vi "DIALOG_Class Selection.vi"(7 "Action":T3=enum."Class For Node", 8 "Error In":errorcluster, 9 "User VI Ref":refnum<vi>, 10 "Class Name In":string, 11 "Classes":T4(array[cluster])=[{"Class Info"={"Unique ID string"="1", "Parent ID string"="", "Class Name (unlocalized)"="Application", "Class Name (localized)"="Application"}, "Class Heirarchy"="Application", "Class Type"=enum."Base", "Indent"=0}, {"Class Info"={"Unique ID string"="98", "Parent ID string"="", "Class Name (unlocalized)"="CopyConflict", "Class Name (localized)"="CopyConflict"}, "Class Heirarchy"="CopyConflict", "Class Type"=enum."Private", "Indent"=0}, {"Class Info"={"Unique ID string"="99", "Parent ID string"="", "Class Name (unlocalized)"="CopyExpert", "Class Name (localized)"="CopyExpert"}, "Class Heirarchy"="CopyExpert", "Class Type"=enum."Private", "Indent"=0}, {"Class Info"={"Unique ID string"="97", "Parent ID string"="", "Class Name (unlocalized)"="CopyItem", "Class Name (localized)"="CopyItem"}, "Class Heirarchy"="CopyItem", "Class Type"=enum."Private", "Indent"=0}, {"Class Info"={"Unique ID string"="94", "Parent ID string"="", "Class Name (unlocalized)"="CopyOperation", "Class Name (localized)"="CopyOperation"}, "Class Heirarchy"="CopyOperation", "Class Type"=enum."Private", "Indent"=0}, {"Class Info"={"Unique ID string"="3", "Parent ID string"="", "Class Name (unlocalized)"="Generic", "Class Name (localized)"="Generic"}, "Class Heirarchy"="Generic", "Class Type"=enum."Base", "Indent"=0}, {"Class Info"={"Unique ID string"="131", "Parent ID string"="3", "Class Name (unlocalized)"="Bus", "Class Name (localized)"="Bus"}, "Class Heirarchy"="Generic.Bus", "Class Type"=enum."Base", "Indent"=1}, {"Class Info"={"Unique ID string"="56", "Parent ID string"="3", "Class Name (unlocalized)"="ConnectorPane", "Class Name (localized)"="ConnectorPane"}, "Class Heirarchy"="Generic.ConnectorPane", "Class Type"=enum."Scripting", "Indent"=1}, {"Class Info"={"Unique ID string"="38", "Parent ID string"="3", "Class Name (unlocalized)"="Cursor", "Class Name (localized)"="Cursor"}, "Class Heirarchy"="Generic.Cursor", "Class Type"=enum."Base", "Indent"=1}, {"Class Info"={"Unique ID string"="16479", "Parent ID string"="3", "Class Name (unlocalized)"="FlatSequenceFrame", "Class Name (localized)"="FlatSequenceFrame"}, "Class Heirarchy"="Generic.FlatSequenceFrame", "Class Type"=enum."Scripting", "Indent"=1}, {"Class Info"={"Unique ID string"="16494", "Parent ID string"="16479", "Class Name (unlocalized)"="TimeSequenceFrame", "Class Name (localized)"="TimeSequenceFrame"}, "Class Heirarchy"="Generic.FlatSequenceFrame.TimeSequenceFrame", "Class Type"=enum."Scripting", "Indent"=2}, {"Class Info"={"Unique ID string"="36", "Parent ID string"="3", "Class Name (unlocalized)"="GObject", "Class Name (localized)"="GObject"}, "Class Heirarchy"="Generic.GObject", "Class Type"=enum."Base", "Indent"=1}, {"Class Info"={"Unique ID string"="16503", "Parent ID string"="36", "Class Name (unlocalized)"="AbstractDiagram", "Class Name (localized)"="AbstractDiagram"}, "Class Heirarchy"="Generic.GObject.AbstractDiagram", "Class Type"=enum."Scripting", "Indent"=2}, {"Class Info"={"Unique ID string"="16384", "Parent ID string"="16503", "Class Name (unlocalized)"="Diagram", "Class Name (localized)"="Diagram"}, "Class Heirarchy"="Generic.GObject.AbstractDiagram.Diagram", "Class Type"=enum."Scripting", "Indent"=3}, {"Class Info"={"Unique ID string"="16473", "Parent ID string"="16384", "Class Name (unlocalized)"="CompanionDiagram", "Class Name (localized)"="CompanionDiagram"}, "Class Heirarchy"="Generic.GObject.AbstractDiagram.Diagram.CompanionDiagram", "Class Type"=enum."Scripting", "Indent"=4}, {"Class Info"={"Unique ID string"="16489", "Parent ID string"="16384", "Class Name (unlocalized)"="SDF Companion Diagram", "Class Name (localized)"="SDF Companion Diagram"}, "Class Heirarchy"="Generic.GObject.AbstractDiagram.Diagram.SDF Companion Diagram", "Class Type"=enum."Scripting", "Indent"=4}, {"Class Info"={"Unique ID string"="16488", "Parent ID string"="16384", "Class Name (unlocalized)"="SDFDiagram", "Class Name (localized)"="SDFDiagram"}, "Class Heirarchy"="Generic.GObject.AbstractDiagram.Diagram.SDFDiagram", "Class Type"=enum."Scripting", "Indent"=4}, {"Class Info"={"Unique ID string"="16511", "Parent ID string"="16384", "Class Name (unlocalized)"="ScDiagram", "Class Name (localized)"="ScDiagram"}, "Class Heirarchy"="Generic.GObject.AbstractDiagram.Diagram.ScDiagram", "Class Type"=enum."Scripting", "Indent"=4}, {"Class Info"={"Unique ID string"="16472", "Parent ID string"="16384", "Class Name (unlocalized)"="SimDiagram", "Class Name (localized)"="SimDiagram"}, "Class Heirarchy"="Generic.GObject.AbstractDiagram.Diagram.SimDiagram", "Class Type"=enum."Scripting", "Indent"=4}, {"Class Info"={"Unique ID string"="16423", "Parent ID string"="16384", "Class Name (unlocalized)"="TopLevelDiagram", "Class Name (localized)"="TopLevelDiagram"}, "Class Heirarchy"="Generic.GObject.AbstractDiagram.Diagram.TopLevelDiagram", "Class Type"=enum."Scripting", "Indent"=4}, {"Class Info"={"Unique ID string"="16502", "Parent ID string"="16503", "Class Name (unlocalized)"="MathDiagram", "Class Name (localized)"="MathDiagram"}, "Class Heirarchy"="Generic.GObject.AbstractDiagram.MathDiagram", "Class Type"=enum."Scripting", "Indent"=3}, {"Class Info"={"Unique ID string"="16386", "Parent ID string"="36", "Class Name (unlocalized)"="Constant", "Class Name (localized)"="Constant"}, "Class Heirarchy"="Generic.GObject.Constant", "Class Type"=enum."Scripting", "Indent"=2}, {"Class Info"={"Unique ID string"="16461", "Parent ID string"="16386", "Class Name (unlocalized)"="AbsTimeConstant", "Class Name (localized)"="AbsTimeConstant"}, "Class Heirarchy"="Generic.GObject.Constant.AbsTimeConstant", "Class Type"=enum."Scripting", "Indent"=3}, {"Class Info"={"Unique ID string"="16388", "Parent ID string"="16386", "Class Name (unlocalized)"="ArrayConstant", "Class Name (localized)"="ArrayConstant"}, "Class Heirarchy"="Generic.GObject.Constant.ArrayConstant", "Class Type"=enum."Scripting", "Indent"=3}, {"Class Info"={"Unique ID string"="16422", "Parent ID string"="16386", "Class Name (unlocalized)"="BooleanConstant", "Class Name (localized)"="BooleanConstant"}, "Class Heirarchy"="Generic.GObject.Constant.BooleanConstant", "Class Type"=enum."Scripting", "Indent"=3}, {"Class Info"={"Unique ID string"="16393", "Parent ID string"="16386", "Class Name (unlocalized)"="ClusterConstant", "Class Name (localized)"="ClusterConstant"}, "Class Heirarchy"="Generic.GObject.Constant.ClusterConstant", "Class Type"=enum."Scripting", "Indent"=3}, {"Class Info"={"Unique ID string"="16450", "Parent ID string"="16386", "Class Name (unlocalized)"="ColorBoxConstant", "Class Name (localized)"="ColorBoxConstant"}, "Class Heirarchy"="Generic.GObject.Constant.ColorBoxConstant", "Class Type"=enum."Scripting", "Indent"=3}, {"Class Info"={"Unique ID string"="16394", "Parent ID string"="16386", "Class Name (unlocalized)"="FixedConstant", "Class Name (localized)"="FixedConstant"}, "Class Heirarchy"="Generic.GObject.Constant.FixedConstant", "Class Type"=enum."Scripting", "Indent"=3}, {"Class Info"={"Unique ID string"="16445", "Parent ID string"="16386", "Class Name (unlocalized)"="IONameConstant", "Class Name (localized)"="IONameConstant"}, "Class Heirarchy"="Generic.GObject.Constant.IONameConstant", "Class Type"=enum."Scripting", "Indent"=3}, {"Class Info"={"Unique ID string"="16447", "Parent ID string"="16445", "Class Name (unlocalized)"="DAQChannelNameConstant", "Class Name (localized)"="DAQChannelNameConstant"}, "Class Heirarchy"="Generic.GObject.Constant.IONameConstant.DAQChannelNameConstant", "Class Type"=enum."Scripting", "Indent"=4}, {"Class Info"={"Unique ID string"="16457", "Parent ID string"="16445", "Class Name (unlocalized)"="DAQmxNameConstant", "Class Name (localized)"="DAQmxNameConstant"}, "Class Heirarchy"="Generic.GObject.Constant.IONameConstant.DAQmxNameConstant", "Class Type"=enum."Scripting", "Indent"=4}, {"Class Info"={"Unique ID string"="16446", "Parent ID string"="16445", "Class Name (unlocalized)"="DSCTagConstant", "Class Name (localized)"="DSCTagConstant"}, "Class Heirarchy"="Generic.GObject.Constant.IONameConstant.DSCTagConstant", "Class Type"=enum."Scripting", "Indent"=4}, {"Class Info"={"Unique ID string"="16470", "Parent ID string"="16445", "Class Name (unlocalized)"="GenClassTagFlatRefConstant", "Class Name (localized)"="GenClassTagFlatRefConstant"}, "Class Heirarchy"="Generic.GObject.Constant.IONameConstant.GenClassTagFlatRefConstant", "Class Type"=enum."Scripting", "Indent"=4}, {"Class Info"={"Unique ID string"="16460", "Parent ID string"="16445", "Class Name (unlocalized)"="GenClassTagRefConstant", "Class Name (localized)"="GenClassTagRefConstant"}, "Class Heirarchy"="Generic.GObject.Constant.IONameConstant.GenClassTagRefConstant", "Class Type"=enum."Scripting", "Indent"=4}, {"Class Info"={"Unique ID string"="16449", "Parent ID string"="16445", "Class Name (unlocalized)"="IVILogicalNameConstant", "Class Name (localized)"="IVILogicalNameConstant"}, "Class Heirarchy"="Generic.GObject.Constant.IONameConstant.IVILogicalNameConstant", "Class Type"=enum."Scripting", "Indent"=4}, {"Class Info"={"Unique ID string"="16448", "Parent ID string"="16445", "Class Name (unlocalized)"="VISAResourceNameConstant", "Class Name (localized)"="VISAResourceNameConstant"}, "Class Heirarchy"="Generic.GObject.Constant.IONameConstant.VISAResourceNameConstant", "Class Type"=enum."Scripting", "Indent"=4}, {"Class Info"={"Unique ID string"="16501", "Parent ID string"="16386", "Class Name (unlocalized)"="LabVIEWClassConstant", "Class Name (localized)"="LabVIEWClassConstant"}, "Class Heirarchy"="Generic.GObject.Constant.LabVIEWClassConstant", "Class Type"=enum."Scripting", "Indent"=3}, {"Class Info"={"Unique ID string"="16553", "Parent ID string"="16386", "Class Name (unlocalized)"="MapConstant", "Class Name (localized)"="MapConstant"}, "Class Heirarchy"="Generic.GObject.Constant.MapConstant", "Class Type"=enum."Scripting", "Indent"=3}, {"Class Info"={"Unique ID string"="16389", "Parent ID string"="16386", "Class Name (unlocalized)"="NumericConstant", "Class Name (localized)"="NumericConstant"}, "Class Heirarchy"="Generic.GObject.Constant.NumericConstant", "Class Type"=enum."Scripting", "Indent"=3}, {"Class Info"={"Unique ID string"="16390", "Parent ID string"="16389", "Class Name (unlocalized)"="DigitalNumericConstant", "Class Name (localized)"="DigitalNumericConstant"}, "Class Heirarchy"="Generic.GObject.Constant.NumericConstant.DigitalNumericConstant", "Class Type"=enum."Scripting", "Indent"=4}, {"Class Info"={"Unique ID string"="16391", "Parent ID string"="16389", "Class Name (unlocalized)"="NamedNumericConstant", "Class Name (localized)"="NamedNumericConstant"}, "Class Heirarchy"="Generic.GObject.Constant.NumericConstant.NamedNumericConstant", "Class Type"=enum."Scripting", "Indent"=4}, {"Class Info"={"Unique ID string"="16425", "Parent ID string"="16391", "Class Name (unlocalized)"="EnumConstant", "Class Name (localized)"="EnumConstant"}, "Class Heirarchy"="Generic.GObject.Constant.NumericConstant.NamedNumericConstant.EnumConstant", "Class Type"=enum."Scripting", "Indent"=5}, {"Class Info"={"Unique ID string"="16424", "Parent ID string"="16391", "Class Name (unlocalized)"="RingConstant", "Class Name (localized)"="RingConstant"}, "Class Heirarchy"="Generic.GObject.Constant.NumericConstant.NamedNumericConstant.RingConstant", "Class Type"=enum."Scripting", "Indent"=5}, {"Class Info"={"Unique ID string"="16387", "Parent ID string"="16386", "Class Name (unlocalized)"="PathConstant", "Class Name (localized)"="PathConstant"}, "Class Heirarchy"="Generic.GObject.Constant.PathConstant", "Class Type"=enum."Scripting", "Indent"=3}, {"Class Info"={"Unique ID string"="16482", "Parent ID string"="16386", "Class Name (unlocalized)"="RefNumConstant", "Class Name (localized)"="RefNumConstant"}, "Class Heirarchy"="Generic.GObject.Constant.RefNumConstant", "Class Type"=enum."Scripting", "Indent"=3}, {"Class Info"={"Unique ID string"="16452", "Parent ID string"="16482", "Class Name (unlocalized)"="ClassSpecifierConstant", "Class Name (localized)"="ClassSpecifierConstant"}, "Class Heirarchy"="Generic.GObject.Constant.RefNumConstant.ClassSpecifierConstant", "Class Type"=enum."Scripting", "Indent"=4}, {"Class Info"={"Unique ID string"="16529", "Parent ID string"="16482", "Class Name (unlocalized)"="GenClassRefConst", "Class Name (localized)"="GenClassRefConst"}, "Class Heirarchy"="Generic.GObject.Constant.RefNumConstant.GenClassRefConst", "Class Type"=enum."Scripting", "Indent"=4}, {"Class Info"={"Unique ID string"="16538", "Parent ID string"="16482", "Class Name (unlocalized)"="TypedRefNumConstant", "Class Name (localized)"="TypedRefNumConstant"}, "Class Heirarchy"="Generic.GObject.Constant.RefNumConstant.TypedRefNumConstant", "Class Type"=enum."Scripting", "Indent"=4}, {"Class Info"={"Unique ID string"="16539", "Parent ID string"="16538", "Class Name (unlocalized)"="DataValRefNumConstant", "Class Name (localized)"="DataValRefNumConstant"}, "Class Heirarchy"="Generic.GObject.Constant.RefNumConstant.TypedRefNumConstant.DataValRefNumConstant", "Class Type"=enum."Scripting", "Indent"=5}, {"Class Info"={"Unique ID string"="16552", "Parent ID string"="16386", "Class Name (unlocalized)"="SetConstant", "Class Name (localized)"="SetConstant"}, "Class Heirarchy"="Generic.GObject.Constant.SetConstant", "Class Type"=enum."Scripting", "Indent"=3}, {"Class Info"={"Unique ID string"="16392", "Parent ID string"="16386", "Class Name (unlocalized)"="StringConstant", "Class Name (localized)"="StringConstant"}, "Class Heirarchy"="Generic.GObject.Constant.StringConstant", "Class Type"=enum."Scripting", "Indent"=3}, {"Class Info"={"Unique ID string"="16466", "Parent ID string"="16392", "Class Name (unlocalized)"="ComboBoxConstant", "Class Name (localized)"="ComboBoxConstant"}, "Class Heirarchy"="Generic.GObject.Constant.StringConstant.ComboBoxConstant", "Class Type"=enum."Scripting", "Indent"=4}, {"Class Info"={"Unique ID string"="6", "Parent ID string"="36", "Class Name (unlocalized)"="Control", "Class Name (localized)"="Control"}, "Class Heirarchy"="Generic.GObject.Control", "Class Type"=enum."Base", "Indent"=2}, {"Class Info"={"Unique ID string"="60", "Parent ID string"="6", "Class Name (unlocalized)"="AbsTime", "Class Name (localized)"="AbsTime"}, "Class Heirarchy"="Generic.GObject.Control.AbsTime", "Class Type"=enum."Base", "Indent"=3}, {"Class Info"={"Unique ID string"="16", "Parent ID string"="6", "Class Name (unlocalized)"="ActiveXContainer", "Class Name (localized)"="ActiveXContainer"}, "Class Heirarchy"="Generic.GObject.Control.ActiveXContainer", "Class Type"=enum."Base", "Indent"=3}, {"Class Info"={"Unique ID string"="14", "Parent ID string"="6", "Class Name (unlocalized)"="Array", "Class Name (localized)"="Array"}, "Class Heirarchy"="Generic.GObject.Control.Array", "Class Type"=enum."Base", "Indent"=3}, {"Class Info"={"Unique ID string"="8", "Parent ID string"="6", "Class Name (unlocalized)"="Boolean", "Class Name (localized)"="Boolean"}, "Class Heirarchy"="Generic.GObject.Control.Boolean", "Class Type"=enum."Base", "Indent"=3}, {"Class Info"={"Unique ID string"="30", "Parent ID string"="6", "Class Name (unlocalized)"="Cluster", "Class Name (localized)"="Cluster"}, "Class Heirarchy"="Generic.GObject.Control.Cluster", "Class Type"=enum."Base", "Indent"=3}, {"Class Info"={"Unique ID string"="72", "Parent ID string"="30", "Class Name (unlocalized)"="RadioButtonsControl", "Class Name (localized)"="RadioButtonsControl"}, "Class Heirarchy"="Generic.GObject.Control.Cluster.RadioButtonsControl", "Class Type"=enum."Base", "Indent"=4}, {"Class Info"={"Unique ID string"="7", "Parent ID string"="6", "Class Name (unlocalized)"="ColorBox", "Class Name (localized)"="ColorBox"}, "Class Heirarchy"="Generic.GObject.Control.ColorBox", "Class Type"=enum."Base", "Indent"=3}, {"Class Info"={"Unique ID string"="61", "Parent ID string"="6", "Class Name (unlocalized)"="DigitalTable", "Class Name (localized)"="DigitalTable"}, "Class Heirarchy"="Generic.GObject.Control.DigitalTable", "Class Type"=enum."Base", "Indent"=3}, {"Class Info"={"Unique ID string"="22", "Parent ID string"="6", "Class Name (unlocalized)"="GraphChart", "Class Name (localized)"="GraphChart"}, "Class Heirarchy"="Generic.GObject.Control.GraphChart", "Class Type"=enum."Base", "Indent"=3}, {"Class Info"={"Unique ID string"="25", "Parent ID string"="22", "Class Name (unlocalized)"="IntensityChart", "Class Name (localized)"="IntensityChart"}, "Class Heirarchy"="Generic.GObject.Control.GraphChart.IntensityChart", "Class Type"=enum."Base", "Indent"=4}, {"Class Info"={"Unique ID string"="26", "Parent ID string"="22", "Class Name (unlocalized)"="IntensityGraph", "Class Name (localized)"="IntensityGraph"}, "Class Heirarchy"="Generic.GObject.Control.GraphChart.IntensityGraph", "Class Type"=enum."Base", "Indent"=4}, {"Class Info"={"Unique ID string"="92", "Parent ID string"="22", "Class Name (unlocalized)"="MixedSignalGraph", "Class Name (localized)"="MixedSignalGraph"}, "Class Heirarchy"="Generic.GObject.Control.GraphChart.MixedSignalGraph", "Class Type"=enum."Base", "Indent"=4}, {"Class Info"={"Unique ID string"="23", "Parent ID string"="22", "Class Name (unlocalized)"="WaveformChart", "Class Name (localized)"="WaveformChart"}, "Class Heirarchy"="Generic.GObject.Control.GraphChart.WaveformChart", "Class Type"=enum."Base", "Indent"=4}, {"Class Info"={"Unique ID string"="24", "Parent ID string"="22", "Class Name (unlocalized)"="WaveformGraph", "Class Name (localized)"="WaveformGraph"}, "Class Heirarchy"="Generic.GObject.Control.GraphChart.WaveformGraph", "Class Type"=enum."Base", "Indent"=4}, {"Class Info"={"Unique ID string"="121", "Parent ID string"="24", "Class Name (unlocalized)"="DigitalGraph", "Class Name (localized)"="DigitalGraph"}, "Class Heirarchy"="Generic.GObject.Control.GraphChart.WaveformGraph.DigitalGraph", "Class Type"=enum."Base", "Indent"=5}, {"Class Info"={"Unique ID string"="83", "Parent ID string"="24", "Class Name (unlocalized)"="XYGraph", "Class Name (localized)"="XYGraph"}, "Class Heirarchy"="Generic.GObject.Control.GraphChart.WaveformGraph.XYGraph", "Class Type"=enum."Base", "Indent"=5}, {"Class Info"={"Unique ID string"="28", "Parent ID string"="6", "Class Name (unlocalized)"="IOName", "Class Name (localized)"="IOName"}, "Class Heirarchy"="Generic.GObject.Control.IOName", "Class Type"=enum."Base", "Indent"=3}, {"Class Info"={"Unique ID string"="49", "Parent ID string"="28", "Class Name (unlocalized)"="DAQChannelName", "Class Name (localized)"="DAQChannelName"}, "Class Heirarchy"="Generic.GObject.Control.IOName.DAQChannelName", "Class Type"=enum."Base", "Indent"=4}, {"Class Info"={"Unique ID string"="57", "Parent ID string"="28", "Class Name (unlocalized)"="DAQmxName", "Class Name (localized)"="DAQmxName"}, "Class Heirarchy"="Generic.GObject.Control.IOName.DAQmxName", "Class Type"=enum."Base", "Indent"=4}, {"Class Info"={"Unique ID string"="48", "Parent ID string"="28", "Class Name (unlocalized)"="DSCTag", "Class Name (localized)"="DSCTag"}, "Class Heirarchy"="Generic.GObject.Control.IOName.DSCTag", "Class Type"=enum."Base", "Indent"=4}, {"Class Info"={"Unique ID string"="122", "Parent ID string"="28", "Class Name (unlocalized)"="GenClassTagFlatRef", "Class Name (localized)"="GenClassTagFlatRef"}, "Class Heirarchy"="Generic.GObject.Control.IOName.GenClassTagFlatRef", "Class Type"=enum."Base", "Indent"=4}, {"Class Info"={"Unique ID string"="67", "Parent ID string"="28", "Class Name (unlocalized)"="GenClassTagRef", "Class Name (localized)"="GenClassTagRef"}, "Class Heirarchy"="Generic.GObject.Control.IOName.GenClassTagRef", "Class Type"=enum."Base", "Indent"=4}, {"Class Info"={"Unique ID string"="51", "Parent ID string"="28", "Class Name (unlocalized)"="IVILogicalName", "Class Name (localized)"="IVILogicalName"}, "Class Heirarchy"="Generic.GObject.Control.IOName.IVILogicalName", "Class Type"=enum."Base", "Indent"=4}, {"Class Info"={"Unique ID string"="50", "Parent ID string"="28", "Class Name (unlocalized)"="VISAResourceName", "Class Name (localized)"="VISAResourceName"}, "Class Heirarchy"="Generic.GObject.Control.IOName.VISAResourceName", "Class Type"=enum."Base", "Indent"=4}, {"Class Info"={"Unique ID string"="10", "Parent ID string"="6", "Class Name (unlocalized)"="LVVariant", "Class Name (localized)"="LVVariant"}, "Class Heirarchy"="Generic.GObject.Control.LVVariant", "Class Type"=enum."Base", "Indent"=3}, {"Class Info"={"Unique ID string"="102", "Parent ID string"="6", "Class Name (unlocalized)"="LabVIEWClassControl", "Class Name (localized)"="LabVIEWClassControl"}, "Class Heirarchy"="Generic.GObject.Control.LabVIEWClassControl", "Class Type"=enum."Base", "Indent"=3}, {"Class Info"={"Unique ID string"="12", "Parent ID string"="6", "Class Name (unlocalized)"="ListBox", "Class Name (localized)"="ListBox"}, "Class Heirarchy"="Generic.GObject.Control.ListBox", "Class Type"=enum."Base", "Indent"=3}, {"Class Info"={"Unique ID string"="137", "Parent ID string"="6", "Class Name (unlocalized)"="Map", "Class Name (localized)"="Map"}, "Class Heirarchy"="Generic.GObject.Control.Map", "Class Type"=enum."Base", "Indent"=3}, {"Class Info"={"Unique ID string"="127", "Parent ID string"="6", "Class Name (unlocalized)"="MixedCheckbox", "Class Name (localized)"="MixedCheckbox"}, "Class Heirarchy"="Generic.GObject.Control.MixedCheckbox", "Class Type"=enum."Base", "Indent"=3}, {"Class Info"={"Unique ID string"="130", "Parent ID string"="6", "Class Name (unlocalized)"="MultiSegmentPipe", "Class Name (localized)"="MultiSegmentPipe"}, "Class Heirarchy"="Generic.GObject.Control.MultiSegmentPipe", "Class Type"=enum."Base", "Indent"=3}, {"Class Info"={"Unique ID string"="46", "Parent ID string"="6", "Class Name (unlocalized)"="MulticolumnListbox", "Class Name (localized)"="MulticolumnListbox"}, "Class Heirarchy"="Generic.GObject.Control.MulticolumnListbox", "Class Type"=enum."Base", "Indent"=3}, {"Class Info"={"Unique ID string"="17", "Parent ID string"="6", "Class Name (unlocalized)"="Numeric", "Class Name (localized)"="Numeric"}, "Class Heirarchy"="Generic.GObject.Control.Numeric", "Class Type"=enum."Base", "Indent"=3}, {"Class Info"={"Unique ID string"="20", "Parent ID string"="17", "Class Name (unlocalized)"="ColorRamp", "Class Name (localized)"="ColorRamp"}, "Class Heirarchy"="Generic.GObject.Control.Numeric.ColorRamp", "Class Type"=enum."Base", "Indent"=4}, {"Class Info"={"Unique ID string"="18", "Parent ID string"="17", "Class Name (unlocalized)"="Digital", "Class Name (localized)"="Digital"}, "Class Heirarchy"="Generic.GObject.Control.Numeric.Digital", "Class Type"=enum."Base", "Indent"=4}, {"Class Info"={"Unique ID string"="19", "Parent ID string"="17", "Class Name (unlocalized)"="NamedNumeric", "Class Name (localized)"="NamedNumeric"}, "Class Heirarchy"="Generic.GObject.Control.Numeric.NamedNumeric", "Class Type"=enum."Base", "Indent"=4}, {"Class Info"={"Unique ID string"="35", "Parent ID string"="19", "Class Name (unlocalized)"="Enum", "Class Name (localized)"="Enum"}, "Class Heirarchy"="Generic.GObject.Control.Numeric.NamedNumeric.Enum", "Class Type"=enum."Base", "Indent"=5}, {"Class Info"={"Unique ID string"="34", "Parent ID string"="19", "Class Name (unlocalized)"="Ring", "Class Name (localized)"="Ring"}, "Class Heirarchy"="Generic.GObject.Control.Numeric.NamedNumeric.Ring", "Class Type"=enum."Base", "Indent"=5}, {"Class Info"={"Unique ID string"="33", "Parent ID string"="17", "Class Name (unlocalized)"="NumericWithScale", "Class Name (localized)"="NumericWithScale"}, "Class Heirarchy"="Generic.GObject.Control.Numeric.NumericWithScale", "Class Type"=enum."Base", "Indent"=4}, {"Class Info"={"Unique ID string"="32", "Parent ID string"="33", "Class Name (unlocalized)"="Knob", "Class Name (localized)"="Knob"}, "Class Heirarchy"="Generic.GObject.Control.Numeric.NumericWithScale.Knob", "Class Type"=enum."Base", "Indent"=5}, {"Class Info"={"Unique ID string"="21", "Parent ID string"="33", "Class Name (unlocalized)"="Slide", "Class Name (localized)"="Slide"}, "Class Heirarchy"="Generic.GObject.Control.Numeric.NumericWithScale.Slide", "Class Type"=enum."Base", "Indent"=5}, {"Class Info"={"Unique ID string"="53", "Parent ID string"="6", "Class Name (unlocalized)"="PageSelector", "Class Name (localized)"="PageSelector"}, "Class Heirarchy"="Generic.GObject.Control.PageSelector", "Class Type"=enum."Base", "Indent"=3}, {"Class Info"={"Unique ID string"="55", "Parent ID string"="53", "Class Name (unlocalized)"="TabControl", "Class Name (localized)"="TabControl"}, "Class Heirarchy"="Generic.GObject.Control.PageSelector.TabControl", "Class Type"=enum."Base", "Indent"=4}, {"Class Info"={"Unique ID string"="11", "Parent ID string"="6", "Class Name (unlocalized)"="Path", "Class Name (localized)"="Path"}, "Class Heirarchy"="Generic.GObject.Control.Path", "Class Type"=enum."Base", "Indent"=3}, {"Class Info"={"Unique ID string"="15", "Parent ID string"="6", "Class Name (unlocalized)"="Picture", "Class Name (localized)"="Picture"}, "Class Heirarchy"="Generic.GObject.Control.Picture", "Class Type"=enum."Base", "Indent"=3}, {"Class Info"={"Unique ID string"="78", "Parent ID string"="6", "Class Name (unlocalized)"="Pixmap", "Class Name (localized)"="Pixmap"}, "Class Heirarchy"="Generic.GObject.Control.Pixmap", "Class Type"=enum."Base", "Indent"=3}, {"Class Info"={"Unique ID string"="70", "Parent ID string"="6", "Class Name (unlocalized)"="PlugInControl", "Class Name (localized)"="PlugInControl"}, "Class Heirarchy"="Generic.GObject.Control.PlugInControl", "Class Type"=enum."Base", "Indent"=3}, {"Class Info"={"Unique ID string"="71", "Parent ID string"="6", "Class Name (unlocalized)"="PlugInDDODummyContainer", "Class Name (localized)"="PlugInDDODummyContainer"}, "Class Heirarchy"="Generic.GObject.Control.PlugInDDODummyContainer", "Class Type"=enum."Base", "Indent"=3}, {"Class Info"={"Unique ID string"="9", "Parent ID string"="6", "Class Name (unlocalized)"="RefNum", "Class Name (localized)"="RefNum"}, "Class Heirarchy"="Generic.GObject.Control.RefNum", "Class Type"=enum."Base", "Indent"=3}, {"Class Info"={"Unique ID string"="68", "Parent ID string"="9", "Class Name (unlocalized)"="GenClassRef", "Class Name (localized)"="GenClassRef"}, "Class Heirarchy"="Generic.GObject.Control.RefNum.GenClassRef", "Class Type"=enum."Base", "Indent"=4}, {"Class Info"={"Unique ID string"="59", "Parent ID string"="9", "Class Name (unlocalized)"="LVObjectRefNum", "Class Name (localized)"="LVObjectRefNum"}, "Class Heirarchy"="Generic.GObject.Control.RefNum.LVObjectRefNum", "Class Type"=enum."Base", "Indent"=4}, {"Class Info"={"Unique ID string"="58", "Parent ID string"="59", "Class Name (unlocalized)"="VIRefNum", "Class Name (localized)"="VIRefNum"}, "Class Heirarchy"="Generic.GObject.Control.RefNum.LVObjectRefNum.VIRefNum", "Class Type"=enum."Base", "Indent"=5}, {"Class Info"={"Unique ID string"="44", "Parent ID string"="9", "Class Name (unlocalized)"="TypedRefNum", "Class Name (localized)"="TypedRefNum"}, "Class Heirarchy"="Generic.GObject.Control.RefNum.TypedRefNum", "Class Type"=enum."Base", "Indent"=4}, {"Class Info"={"Unique ID string"="135", "Parent ID string"="44", "Class Name (unlocalized)"="DataValRefNum", "Class Name (localized)"="DataValRefNum"}, "Class Heirarchy"="Generic.GObject.Control.RefNum.TypedRefNum.DataValRefNum", "Class Type"=enum."Base", "Indent"=5}, {"Class Info"={"Unique ID string"="100", "Parent ID string"="6", "Class Name (unlocalized)"="SceneGraphDisplay", "Class Name (localized)"="SceneGraphDisplay"}, "Class Heirarchy"="Generic.GObject.Control.SceneGraphDisplay", "Class Type"=enum."Base", "Indent"=3}, {"Class Info"={"Unique ID string"="90", "Parent ID string"="6", "Class Name (unlocalized)"="Scrollbar", "Class Name (localized)"="Scrollbar"}, "Class Heirarchy"="Generic.GObject.Control.Scrollbar", "Class Type"=enum."Base", "Indent"=3}, {"Class Info"={"Unique ID string"="136", "Parent ID string"="6", "Class Name (unlocalized)"="Set", "Class Name (localized)"="Set"}, "Class Heirarchy"="Generic.GObject.Control.Set", "Class Type"=enum."Base", "Indent"=3}, {"Class Info"={"Unique ID string"="27", "Parent ID string"="6", "Class Name (unlocalized)"="String", "Class Name (localized)"="String"}, "Class Heirarchy"="Generic.GObject.Control.String", "Class Type"=enum."Base", "Indent"=3}, {"Class Info"={"Unique ID string"="29", "Parent ID string"="27", "Class Name (unlocalized)"="ComboBox", "Class Name (localized)"="ComboBox"}, "Class Heirarchy"="Generic.GObject.Control.String.ComboBox", "Class Type"=enum."Base", "Indent"=4}, {"Class Info"={"Unique ID string"="132", "Parent ID string"="6", "Class Name (unlocalized)"="StubDDO", "Class Name (localized)"="StubDDO"}, "Class Heirarchy"="Generic.GObject.Control.StubDDO", "Class Type"=enum."Base", "Indent"=3}, {"Class Info"={"Unique ID string"="65", "Parent ID string"="6", "Class Name (unlocalized)"="SubPanel", "Class Name (localized)"="SubPanel"}, "Class Heirarchy"="Generic.GObject.Control.SubPanel", "Class Type"=enum."Base", "Indent"=3}, {"Class Info"={"Unique ID string"="13", "Parent ID string"="6", "Class Name (unlocalized)"="Table", "Class Name (localized)"="Table"}, "Class Heirarchy"="Generic.GObject.Control.Table", "Class Type"=enum."Base", "Indent"=3}, {"Class Info"={"Unique ID string"="66", "Parent ID string"="6", "Class Name (unlocalized)"="TreeControl", "Class Name (localized)"="TreeControl"}, "Class Heirarchy"="Generic.GObject.Control.TreeControl", "Class Type"=enum."Base", "Indent"=3}, {"Class Info"={"Unique ID string"="47", "Parent ID string"="6", "Class Name (unlocalized)"="WaveformData", "Class Name (localized)"="WaveformData"}, "Class Heirarchy"="Generic.GObject.Control.WaveformData", "Class Type"=enum."Base", "Indent"=3}, {"Class Info"={"Unique ID string"="4", "Parent ID string"="36", "Class Name (unlocalized)"="Decoration", "Class Name (localized)"="Decoration"}, "Class Heirarchy"="Generic.GObject.Decoration", "Class Type"=enum."Base", "Indent"=2}, {"Class Info"={"Unique ID string"="5", "Parent ID string"="4", "Class Name (unlocalized)"="Text", "Class Name (localized)"="Text"}, "Class Heirarchy"="Generic.GObject.Decoration.Text", "Class Type"=enum."Base", "Indent"=3}, {"Class Info"={"Unique ID string"="39", "Parent ID string"="5", "Class Name (unlocalized)"="NumericText", "Class Name (localized)"="NumericText"}, "Class Heirarchy"="Generic.GObject.Decoration.Text.NumericText", "Class Type"=enum."Base", "Indent"=4}, {"Class Info"={"Unique ID string"="16459", "Parent ID string"="36", "Class Name (unlocalized)"="FlatSequence", "Class Name (localized)"="FlatSequence"}, "Class Heirarchy"="Generic.GObject.FlatSequence", "Class Type"=enum."Scripting", "Indent"=2}, {"Class Info"={"Unique ID string"="16495", "Parent ID string"="16459", "Class Name (unlocalized)"="TimeFlatSequence", "Class Name (localized)"="TimeFlatSequence"}, "Class Heirarchy"="Generic.GObject.FlatSequence.TimeFlatSequence", "Class Type"=enum."Scripting", "Indent"=3}, {"Class Info"={"Unique ID string"="16480", "Parent ID string"="36", "Class Name (unlocalized)"="FlatSequenceInnerTunnel", "Class Name (localized)"="FlatSequenceInnerTunnel"}, "Class Heirarchy"="Generic.GObject.FlatSequenceInnerTunnel", "Class Type"=enum."Scripting", "Indent"=2}, {"Class Info"={"Unique ID string"="16481", "Parent ID string"="36", "Class Name (unlocalized)"="FlatSequenceOuterTunnel", "Class Name (localized)"="FlatSequenceOuterTunnel"}, "Class Heirarchy"="Generic.GObject.FlatSequenceOuterTunnel", "Class Type"=enum."Scripting", "Indent"=2}, {"Class Info"={"Unique ID string"="16396", "Parent ID string"="36", "Class Name (unlocalized)"="FormulaParameter", "Class Name (localized)"="FormulaParameter"}, "Class Heirarchy"="Generic.GObject.FormulaParameter", "Class Type"=enum."Scripting", "Indent"=2}, {"Class Info"={"Unique ID string"="16500", "Parent ID string"="16396", "Class Name (unlocalized)"="MathScriptNodeParameter", "Class Name (localized)"="MathScriptNodeParameter"}, "Class Heirarchy"="Generic.GObject.FormulaParameter.MathScriptNodeParameter", "Class Type"=enum."Scripting", "Indent"=3}, {"Class Info"={"Unique ID string"="16464", "Parent ID string"="16396", "Class Name (unlocalized)"="ScriptNodeParameter", "Class Name (localized)"="ScriptNodeParameter"}, "Class Heirarchy"="Generic.GObject.FormulaParameter.ScriptNodeParameter", "Class Type"=enum."Scripting", "Indent"=3}, {"Class Info"={"Unique ID string"="16421", "Parent ID string"="36", "Class Name (unlocalized)"="Node", "Class Name (localized)"="Node"}, "Class Heirarchy"="Generic.GObject.Node", "Class Type"=enum."Scripting", "Indent"=2}, {"Class Info"={"Unique ID string"="16402", "Parent ID string"="16421", "Class Name (unlocalized)"="CallByRef", "Class Name (localized)"="CallByRef"}, "Class Heirarchy"="Generic.GObject.Node.CallByRef", "Class Type"=enum."Scripting", "Indent"=3}, {"Class Info"={"Unique ID string"="16451", "Parent ID string"="16421", "Class Name (unlocalized)"="ControlReferenceConstant", "Class Name (localized)"="ControlReferenceConstant"}, "Class Heirarchy"="Generic.GObject.Node.ControlReferenceConstant", "Class Type"=enum."Scripting", "Indent"=3}, {"Class Info"={"Unique ID string"="16522", "Parent ID string"="16421", "Class Name (unlocalized)"="FeedbackNode", "Class Name (localized)"="FeedbackNode"}, "Class Heirarchy"="Generic.GObject.Node.FeedbackNode", "Class Type"=enum."Scripting", "Indent"=3}, {"Class Info"={"Unique ID string"="16409", "Parent ID string"="16421", "Class Name (unlocalized)"="Formula", "Class Name (localized)"="Formula"}, "Class Heirarchy"="Generic.GObject.Node.Formula", "Class Type"=enum."Scripting", "Indent"=3}, {"Class Info"={"Unique ID string"="16504", "Parent ID string"="16409", "Class Name (unlocalized)"="InlineCNode", "Class Name (localized)"="InlineCNode"}, "Class Heirarchy"="Generic.GObject.Node.Formula.InlineCNode", "Class Type"=enum."Scripting", "Indent"=4}, {"Class Info"={"Unique ID string"="16499", "Parent ID string"="16409", "Class Name (unlocalized)"="MathScriptNode", "Class Name (localized)"="MathScriptNode"}, "Class Heirarchy"="Generic.GObject.Node.Formula.MathScriptNode", "Class Type"=enum."Scripting", "Indent"=4}, {"Class Info"={"Unique ID string"="16436", "Parent ID string"="16409", "Class Name (unlocalized)"="ScriptNode", "Class Name (localized)"="ScriptNode"}, "Class Heirarchy"="Generic.GObject.Node.Formula.ScriptNode", "Class Type"=enum."Scripting", "Indent"=4}, {"Class Info"={"Unique ID string"="16400", "Parent ID string"="16421", "Class Name (unlocalized)"="Function", "Class Name (localized)"="Function"}, "Class Heirarchy"="Generic.GObject.Node.Function", "Class Type"=enum."Scripting", "Indent"=3}, {"Class Info"={"Unique ID string"="16437", "Parent ID string"="16400", "Class Name (unlocalized)"="ArrayToCluster", "Class Name (localized)"="ArrayToCluster"}, "Class Heirarchy"="Generic.GObject.Node.Function.ArrayToCluster", "Class Type"=enum."Scripting", "Indent"=4}, {"Class Info"={"Unique ID string"="16429", "Parent ID string"="16400", "Class Name (unlocalized)"="Comparison", "Class Name (localized)"="Comparison"}, "Class Heirarchy"="Generic.GObject.Node.Function.Comparison", "Class Type"=enum."Scripting", "Indent"=4}, {"Class Info"={"Unique ID string"="16535", "Parent ID string"="16429", "Class Name (unlocalized)"="InRangeAndCoerce", "Class Name (localized)"="InRangeAndCoerce"}, "Class Heirarchy"="Generic.GObject.Node.Function.Comparison.InRangeAndCoerce", "Class Type"=enum."Scripting", "Indent"=5}, {"Class Info"={"Unique ID string"="16492", "Parent ID string"="16400", "Class Name (unlocalized)"="FileDialog", "Class Name (localized)"="FileDialog"}, "Class Heirarchy"="Generic.GObject.Node.Function.FileDialog", "Class Type"=enum."Scripting", "Indent"=4}, {"Class Info"={"Unique ID string"="16432", "Parent ID string"="16400", "Class Name (unlocalized)"="FlattenUnflattenString", "Class Name (localized)"="FlattenUnflattenString"}, "Class Heirarchy"="Generic.GObject.Node.Function.FlattenUnflattenString", "Class Type"=enum."Scripting", "Indent"=4}, {"Class Info"={"Unique ID string"="16483", "Parent ID string"="16432", "Class Name (unlocalized)"="FlattenString", "Class Name (localized)"="FlattenString"}, "Class Heirarchy"="Generic.GObject.Node.Function.FlattenUnflattenString.FlattenString", "Class Type"=enum."Scripting", "Indent"=5}, {"Class Info"={"Unique ID string"="16433", "Parent ID string"="16400", "Class Name (unlocalized)"="GPIBReadWrite", "Class Name (localized)"="GPIBReadWrite"}, "Class Heirarchy"="Generic.GObject.Node.Function.GPIBReadWrite", "Class Type"=enum."Scripting", "Indent"=4}, {"Class Info"={"Unique ID string"="16430", "Parent ID string"="16400", "Class Name (unlocalized)"="ReadWriteFile", "Class Name (localized)"="ReadWriteFile"}, "Class Heirarchy"="Generic.GObject.Node.Function.ReadWriteFile", "Class Type"=enum."Scripting", "Indent"=4}, {"Class Info"={"Unique ID string"="16431", "Parent ID string"="16400", "Class Name (unlocalized)"="TypeCast", "Class Name (localized)"="TypeCast"}, "Class Heirarchy"="Generic.GObject.Node.Function.TypeCast", "Class Type"=enum."Scripting", "Indent"=4}, {"Class Info"={"Unique ID string"="16397", "Parent ID string"="16421", "Class Name (unlocalized)"="Global", "Class Name (localized)"="Global"}, "Class Heirarchy"="Generic.GObject.Node.Global", "Class Type"=enum."Scripting", "Indent"=3}, {"Class Info"={"Unique ID string"="16410", "Parent ID string"="16421", "Class Name (unlocalized)"="GrowableFunction", "Class Name (localized)"="GrowableFunction"}, "Class Heirarchy"="Generic.GObject.Node.GrowableFunction", "Class Type"=enum."Scripting", "Indent"=3}, {"Class Info"={"Unique ID string"="16551", "Parent ID string"="16410", "Class Name (unlocalized)"="AssertStructuralTypeMismatchNode", "Class Name (localized)"="AssertStructuralTypeMismatchNode"}, "Class Heirarchy"="Generic.GObject.Node.GrowableFunction.AssertStructuralTypeMismatchNode", "Class Type"=enum."Scripting", "Indent"=4}, {"Class Info"={"Unique ID string"="16411", "Parent ID string"="16410", "Class Name (unlocalized)"="BuildClusterArray", "Class Name (localized)"="BuildClusterArray"}, "Class Heirarchy"="Generic.GObject.Node.GrowableFunction.BuildClusterArray", "Class Type"=enum."Scripting", "Indent"=4}, {"Class Info"={"Unique ID string"="16550", "Parent ID string"="16410", "Class Name (unlocalized)"="BuildMapNode", "Class Name (localized)"="BuildMapNode"}, "Class Heirarchy"="Generic.GObject.Node.GrowableFunction.BuildMapNode", "Class Type"=enum."Scripting", "Indent"=4}, {"Class Info"={"Unique ID string"="16549", "Parent ID string"="16410", "Class Name (unlocalized)"="BuildSetNode", "Class Name (localized)"="BuildSetNode"}, "Class Heirarchy"="Generic.GObject.Node.GrowableFunction.BuildSetNode", "Class Type"=enum."Scripting", "Indent"=4}, {"Class Info"={"Unique ID string"="16476", "Parent ID string"="16410", "Class Name (unlocalized)"="Bundler", "Class Name (localized)"="Bundler"}, "Class Heirarchy"="Generic.GObject.Node.GrowableFunction.Bundler", "Class Type"=enum."Scripting", "Indent"=4}, {"Class Info"={"Unique ID string"="16414", "Parent ID string"="16476", "Class Name (unlocalized)"="BuildArray", "Class Name (localized)"="BuildArray"}, "Class Heirarchy"="Generic.GObject.Node.GrowableFunction.Bundler.BuildArray", "Class Type"=enum."Scripting", "Indent"=5}, {"Class Info"={"Unique ID string"="16415", "Parent ID string"="16476", "Class Name (unlocalized)"="NamedBundler", "Class Name (localized)"="NamedBundler"}, "Class Heirarchy"="Generic.GObject.Node.GrowableFunction.Bundler.NamedBundler", "Class Type"=enum."Scripting", "Indent"=5}, {"Class Info"={"Unique ID string"="16416", "Parent ID string"="16410", "Class Name (unlocalized)"="CIN", "Class Name (localized)"="CIN"}, "Class Heirarchy"="Generic.GObject.Node.GrowableFunction.CIN", "Class Type"=enum."Scripting", "Indent"=4}, {"Class Info"={"Unique ID string"="16417", "Parent ID string"="16410", "Class Name (unlocalized)"="CallLibrary", "Class Name (localized)"="CallLibrary"}, "Class Heirarchy"="Generic.GObject.Node.GrowableFunction.CallLibrary", "Class Type"=enum."Scripting", "Indent"=4}, {"Class Info"={"Unique ID string"="16412", "Parent ID string"="16410", "Class Name (unlocalized)"="CompoundArithmetic", "Class Name (localized)"="CompoundArithmetic"}, "Class Heirarchy"="Generic.GObject.Node.GrowableFunction.CompoundArithmetic", "Class Type"=enum."Scripting", "Indent"=4}, {"Class Info"={"Unique ID string"="16438", "Parent ID string"="16410", "Class Name (unlocalized)"="FormatScanString", "Class Name (localized)"="FormatScanString"}, "Class Heirarchy"="Generic.GObject.Node.GrowableFunction.FormatScanString", "Class Type"=enum."Scripting", "Indent"=4}, {"Class Info"={"Unique ID string"="16413", "Parent ID string"="16410", "Class Name (unlocalized)"="IndexArray", "Class Name (localized)"="IndexArray"}, "Class Heirarchy"="Generic.GObject.Node.GrowableFunction.IndexArray", "Class Type"=enum."Scripting", "Indent"=4}, {"Class Info"={"Unique ID string"="16418", "Parent ID string"="16410", "Class Name (unlocalized)"="ObjectFunction", "Class Name (localized)"="ObjectFunction"}, "Class Heirarchy"="Generic.GObject.Node.GrowableFunction.ObjectFunction", "Class Type"=enum."Scripting", "Indent"=4}, {"Class Info"={"Unique ID string"="16505", "Parent ID string"="16418", "Class Name (unlocalized)"="Constructor", "Class Name (localized)"="Constructor"}, "Class Heirarchy"="Generic.GObject.Node.GrowableFunction.ObjectFunction.Constructor", "Class Type"=enum."Scripting", "Indent"=5}, {"Class Info"={"Unique ID string"="16420", "Parent ID string"="16418", "Class Name (unlocalized)"="Invoke", "Class Name (localized)"="Invoke"}, "Class Heirarchy"="Generic.GObject.Node.GrowableFunction.ObjectFunction.Invoke", "Class Type"=enum."Scripting", "Indent"=5}, {"Class Info"={"Unique ID string"="16419", "Parent ID string"="16418", "Class Name (unlocalized)"="Property", "Class Name (localized)"="Property"}, "Class Heirarchy"="Generic.GObject.Node.GrowableFunction.ObjectFunction.Property", "Class Type"=enum."Scripting", "Indent"=5}, {"Class Info"={"Unique ID string"="16542", "Parent ID string"="16410", "Class Name (unlocalized)"="RegisterForEvents", "Class Name (localized)"="RegisterForEvents"}, "Class Heirarchy"="Generic.GObject.Node.GrowableFunction.RegisterForEvents", "Class Type"=enum."Scripting", "Indent"=4}, {"Class Info"={"Unique ID string"="16477", "Parent ID string"="16410", "Class Name (unlocalized)"="Unbundler", "Class Name (localized)"="Unbundler"}, "Class Heirarchy"="Generic.GObject.Node.GrowableFunction.Unbundler", "Class Type"=enum."Scripting", "Indent"=4}, {"Class Info"={"Unique ID string"="16478", "Parent ID string"="16477", "Class Name (unlocalized)"="NamedUnbundler", "Class Name (localized)"="NamedUnbundler"}, "Class Heirarchy"="Generic.GObject.Node.GrowableFunction.Unbundler.NamedUnbundler", "Class Type"=enum."Scripting", "Indent"=5}, {"Class Info"={"Unique ID string"="16517", "Parent ID string"="16421", "Class Name (unlocalized)"="InPlaceBorderNode", "Class Name (localized)"="InPlaceBorderNode"}, "Class Heirarchy"="Generic.GObject.Node.InPlaceBorderNode", "Class Type"=enum."Scripting", "Indent"=3}, {"Class Info"={"Unique ID string"="16518", "Parent ID string"="16517", "Class Name (unlocalized)"="InPlaceArrayNode", "Class Name (localized)"="InPlaceArrayNode"}, "Class Heirarchy"="Generic.GObject.Node.InPlaceBorderNode.InPlaceArrayNode", "Class Type"=enum."Scripting", "Indent"=4}, {"Class Info"={"Unique ID string"="16530", "Parent ID string"="16517", "Class Name (unlocalized)"="InPlaceArraySplitNode", "Class Name (localized)"="InPlaceArraySplitNode"}, "Class Heirarchy"="Generic.GObject.Node.InPlaceBorderNode.InPlaceArraySplitNode", "Class Type"=enum."Scripting", "Indent"=4}, {"Class Info"={"Unique ID string"="16519", "Parent ID string"="16517", "Class Name (unlocalized)"="InPlaceClusterNode", "Class Name (localized)"="InPlaceClusterNode"}, "Class Heirarchy"="Generic.GObject.Node.InPlaceBorderNode.InPlaceClusterNode", "Class Type"=enum."Scripting", "Indent"=4}, {"Class Info"={"Unique ID string"="16524", "Parent ID string"="16517", "Class Name (unlocalized)"="InPlaceDataValRefNode", "Class Name (localized)"="InPlaceDataValRefNode"}, "Class Heirarchy"="Generic.GObject.Node.InPlaceBorderNode.InPlaceDataValRefNode", "Class Type"=enum."Scripting", "Indent"=4}, {"Class Info"={"Unique ID string"="16521", "Parent ID string"="16517", "Class Name (unlocalized)"="InPlaceElementNode", "Class Name (localized)"="InPlaceElementNode"}, "Class Heirarchy"="Generic.GObject.Node.InPlaceBorderNode.InPlaceElementNode", "Class Type"=enum."Scripting", "Indent"=4}, {"Class Info"={"Unique ID string"="16548", "Parent ID string"="16517", "Class Name (unlocalized)"="InPlaceMapNode", "Class Name (localized)"="InPlaceMapNode"}, "Class Heirarchy"="Generic.GObject.Node.InPlaceBorderNode.InPlaceMapNode", "Class Type"=enum."Scripting", "Indent"=4}, {"Class Info"={"Unique ID string"="16544", "Parent ID string"="16517", "Class Name (unlocalized)"="InPlaceVariantAttributeNode", "Class Name (localized)"="InPlaceVariantAttributeNode"}, "Class Heirarchy"="Generic.GObject.Node.InPlaceBorderNode.InPlaceVariantAttributeNode", "Class Type"=enum."Scripting", "Indent"=4}, {"Class Info"={"Unique ID string"="16520", "Parent ID string"="16517", "Class Name (unlocalized)"="InPlaceVariantNode", "Class Name (localized)"="InPlaceVariantNode"}, "Class Heirarchy"="Generic.GObject.Node.InPlaceBorderNode.InPlaceVariantNode", "Class Type"=enum."Scripting", "Indent"=4}, {"Class Info"={"Unique ID string"="16398", "Parent ID string"="16421", "Class Name (unlocalized)"="Local", "Class Name (localized)"="Local"}, "Class Heirarchy"="Generic.GObject.Node.Local", "Class Type"=enum."Scripting", "Indent"=3}, {"Class Info"={"Unique ID string"="16523", "Parent ID string"="16421", "Class Name (unlocalized)"="MathScriptCallByRef", "Class Name (localized)"="MathScriptCallByRef"}, "Class Heirarchy"="Generic.GObject.Node.MathScriptCallByRef", "Class Type"=enum."Scripting", "Indent"=3}, {"Class Info"={"Unique ID string"="16531", "Parent ID string"="16421", "Class Name (unlocalized)"="SharedVariableDynamicOpen", "Class Name (localized)"="SharedVariableDynamicOpen"}, "Class Heirarchy"="Generic.GObject.Node.SharedVariableDynamicOpen", "Class Type"=enum."Scripting", "Indent"=3}, {"Class Info"={"Unique ID string"="16532", "Parent ID string"="16421", "Class Name (unlocalized)"="SharedVariableDynamicRead", "Class Name (localized)"="SharedVariableDynamicRead"}, "Class Heirarchy"="Generic.GObject.Node.SharedVariableDynamicRead", "Class Type"=enum."Scripting", "Indent"=3}, {"Class Info"={"Unique ID string"="16533", "Parent ID string"="16421", "Class Name (unlocalized)"="SharedVariableDynamicWrite", "Class Name (localized)"="SharedVariableDynamicWrite"}, "Class Heirarchy"="Generic.GObject.Node.SharedVariableDynamicWrite", "Class Type"=enum."Scripting", "Indent"=3}, {"Class Info"={"Unique ID string"="16512", "Parent ID string"="16421", "Class Name (unlocalized)"="SharedVariableNode", "Class Name (localized)"="SharedVariableNode"}, "Class Heirarchy"="Generic.GObject.Node.SharedVariableNode", "Class Type"=enum."Scripting", "Indent"=3}, {"Class Info"={"Unique ID string"="16465", "Parent ID string"="16421", "Class Name (unlocalized)"="StaticVIReference", "Class Name (localized)"="StaticVIReference"}, "Class Heirarchy"="Generic.GObject.Node.StaticVIReference", "Class Type"=enum."Scripting", "Indent"=3}, {"Class Info"={"Unique ID string"="16404", "Parent ID string"="16421", "Class Name (unlocalized)"="Structure", "Class Name (localized)"="Structure"}, "Class Heirarchy"="Generic.GObject.Node.Structure", "Class Type"=enum."Scripting", "Indent"=3}, {"Class Info"={"Unique ID string"="16545", "Parent ID string"="16404", "Class Name (unlocalized)"="ClosureStructureNode", "Class Name (localized)"="ClosureStructureNode"}, "Class Heirarchy"="Generic.GObject.Node.Structure.ClosureStructureNode", "Class Type"=enum."Scripting", "Indent"=4}, {"Class Info"={"Unique ID string"="16516", "Parent ID string"="16404", "Class Name (unlocalized)"="InPlaceElementStructure", "Class Name (localized)"="InPlaceElementStructure"}, "Class Heirarchy"="Generic.GObject.Node.Structure.InPlaceElementStructure", "Class Type"=enum."Scripting", "Indent"=4}, {"Class Info"={"Unique ID string"="16405", "Parent ID string"="16404", "Class Name (unlocalized)"="Loop", "Class Name (localized)"="Loop"}, "Class Heirarchy"="Generic.GObject.Node.Structure.Loop", "Class Type"=enum."Scripting", "Indent"=4}, {"Class Info"={"Unique ID string"="16434", "Parent ID string"="16405", "Class Name (unlocalized)"="ForLoop", "Class Name (localized)"="ForLoop"}, "Class Heirarchy"="Generic.GObject.Node.Structure.Loop.ForLoop", "Class Type"=enum."Scripting", "Indent"=5}, {"Class Info"={"Unique ID string"="16435", "Parent ID string"="16405", "Class Name (unlocalized)"="WhileLoop", "Class Name (localized)"="WhileLoop"}, "Class Heirarchy"="Generic.GObject.Node.Structure.Loop.WhileLoop", "Class Type"=enum."Scripting", "Indent"=5}, {"Class Info"={"Unique ID string"="16467", "Parent ID string"="16435", "Class Name (unlocalized)"="TimedLoop", "Class Name (localized)"="TimedLoop"}, "Class Heirarchy"="Generic.GObject.Node.Structure.Loop.WhileLoop.TimedLoop", "Class Type"=enum."Scripting", "Indent"=6}, {"Class Info"={"Unique ID string"="16406", "Parent ID string"="16404", "Class Name (unlocalized)"="MultiFrameStructure", "Class Name (localized)"="MultiFrameStructure"}, "Class Heirarchy"="Generic.GObject.Node.Structure.MultiFrameStructure", "Class Type"=enum."Scripting", "Indent"=4}, {"Class Info"={"Unique ID string"="16408", "Parent ID string"="16406", "Class Name (unlocalized)"="CaseStructure", "Class Name (localized)"="CaseStructure"}, "Class Heirarchy"="Generic.GObject.Node.Structure.MultiFrameStructure.CaseStructure", "Class Type"=enum."Scripting", "Indent"=5}, {"Class Info"={"Unique ID string"="16487", "Parent ID string"="16406", "Class Name (unlocalized)"="DisableStructure", "Class Name (localized)"="DisableStructure"}, "Class Heirarchy"="Generic.GObject.Node.Structure.MultiFrameStructure.DisableStructure", "Class Type"=enum."Scripting", "Indent"=5}, {"Class Info"={"Unique ID string"="16458", "Parent ID string"="16406", "Class Name (unlocalized)"="EventStructure", "Class Name (localized)"="EventStructure"}, "Class Heirarchy"="Generic.GObject.Node.Structure.MultiFrameStructure.EventStructure", "Class Type"=enum."Scripting", "Indent"=5}, {"Class Info"={"Unique ID string"="16546", "Parent ID string"="16406", "Class Name (unlocalized)"="RaceStructureNode", "Class Name (localized)"="RaceStructureNode"}, "Class Heirarchy"="Generic.GObject.Node.Structure.MultiFrameStructure.RaceStructureNode", "Class Type"=enum."Scripting", "Indent"=5}, {"Class Info"={"Unique ID string"="16407", "Parent ID string"="16406", "Class Name (unlocalized)"="Sequence", "Class Name (localized)"="Sequence"}, "Class Heirarchy"="Generic.GObject.Node.Structure.MultiFrameStructure.Sequence", "Class Type"=enum."Scripting", "Indent"=5}, {"Class Info"={"Unique ID string"="16462", "Parent ID string"="16407", "Class Name (unlocalized)"="ExternalNode", "Class Name (localized)"="ExternalNode"}, "Class Heirarchy"="Generic.GObject.Node.Structure.MultiFrameStructure.Sequence.ExternalNode", "Class Type"=enum."Scripting", "Indent"=6}, {"Class Info"={"Unique ID string"="16474", "Parent ID string"="16404", "Class Name (unlocalized)"="SimulationNode", "Class Name (localized)"="SimulationNode"}, "Class Heirarchy"="Generic.GObject.Node.Structure.SimulationNode", "Class Type"=enum."Scripting", "Indent"=4}, {"Class Info"={"Unique ID string"="16537", "Parent ID string"="16404", "Class Name (unlocalized)"="StatechartStructureNode", "Class Name (localized)"="StatechartStructureNode"}, "Class Heirarchy"="Generic.GObject.Node.Structure.StatechartStructureNode", "Class Type"=enum."Scripting", "Indent"=4}, {"Class Info"={"Unique ID string"="16509", "Parent ID string"="16537", "Class Name (unlocalized)"="ForkNode", "Class Name (localized)"="ForkNode"}, "Class Heirarchy"="Generic.GObject.Node.Structure.StatechartStructureNode.ForkNode", "Class Type"=enum."Scripting", "Indent"=5}, {"Class Info"={"Unique ID string"="16510", "Parent ID string"="16537", "Class Name (unlocalized)"="JoinNode", "Class Name (localized)"="JoinNode"}, "Class Heirarchy"="Generic.GObject.Node.Structure.StatechartStructureNode.JoinNode", "Class Type"=enum."Scripting", "Indent"=5}, {"Class Info"={"Unique ID string"="16507", "Parent ID string"="16537", "Class Name (unlocalized)"="JunctionNode", "Class Name (localized)"="JunctionNode"}, "Class Heirarchy"="Generic.GObject.Node.Structure.StatechartStructureNode.JunctionNode", "Class Type"=enum."Scripting", "Indent"=5}, {"Class Info"={"Unique ID string"="16506", "Parent ID string"="16537", "Class Name (unlocalized)"="RegionNode", "Class Name (localized)"="RegionNode"}, "Class Heirarchy"="Generic.GObject.Node.Structure.StatechartStructureNode.RegionNode", "Class Type"=enum."Scripting", "Indent"=5}, {"Class Info"={"Unique ID string"="16508", "Parent ID string"="16537", "Class Name (unlocalized)"="StateNode", "Class Name (localized)"="StateNode"}, "Class Heirarchy"="Generic.GObject.Node.Structure.StatechartStructureNode.StateNode", "Class Type"=enum."Scripting", "Indent"=5}, {"Class Info"={"Unique ID string"="16490", "Parent ID string"="16404", "Class Name (unlocalized)"="SynchronousDataFlowNode", "Class Name (localized)"="SynchronousDataFlowNode"}, "Class Heirarchy"="Generic.GObject.Node.Structure.SynchronousDataFlowNode", "Class Type"=enum."Scripting", "Indent"=4}, {"Class Info"={"Unique ID string"="16543", "Parent ID string"="16404", "Class Name (unlocalized)"="TargetStructureNode", "Class Name (localized)"="TargetStructureNode"}, "Class Heirarchy"="Generic.GObject.Node.Structure.TargetStructureNode", "Class Type"=enum."Scripting", "Indent"=4}, {"Class Info"={"Unique ID string"="16496", "Parent ID string"="16404", "Class Name (unlocalized)"="TimedSequence", "Class Name (localized)"="TimedSequence"}, "Class Heirarchy"="Generic.GObject.Node.Structure.TimedSequence", "Class Type"=enum."Scripting", "Indent"=4}, {"Class Info"={"Unique ID string"="16401", "Parent ID string"="16421", "Class Name (unlocalized)"="SubVI", "Class Name (localized)"="SubVI"}, "Class Heirarchy"="Generic.GObject.Node.SubVI", "Class Type"=enum."Scripting", "Indent"=3}, {"Class Info"={"Unique ID string"="16526", "Parent ID string"="16401", "Class Name (unlocalized)"="AbstractDynamicDispatch", "Class Name (localized)"="AbstractDynamicDispatch"}, "Class Heirarchy"="Generic.GObject.Node.SubVI.AbstractDynamicDispatch", "Class Type"=enum."Scripting", "Indent"=4}, {"Class Info"={"Unique ID string"="16528", "Parent ID string"="16526", "Class Name (unlocalized)"="CallParentNode", "Class Name (localized)"="CallParentNode"}, "Class Heirarchy"="Generic.GObject.Node.SubVI.AbstractDynamicDispatch.CallParentNode", "Class Type"=enum."Scripting", "Indent"=5}, {"Class Info"={"Unique ID string"="16527", "Parent ID string"="16526", "Class Name (unlocalized)"="DynamicDispatchSubVI", "Class Name (localized)"="DynamicDispatchSubVI"}, "Class Heirarchy"="Generic.GObject.Node.SubVI.AbstractDynamicDispatch.DynamicDispatchSubVI", "Class Type"=enum."Scripting", "Indent"=5}, {"Class Info"={"Unique ID string"="16453", "Parent ID string"="16401", "Class Name (unlocalized)"="ConfNode", "Class Name (localized)"="ConfNode"}, "Class Heirarchy"="Generic.GObject.Node.SubVI.ConfNode", "Class Type"=enum."Scripting", "Indent"=4}, {"Class Info"={"Unique ID string"="16534", "Parent ID string"="16401", "Class Name (unlocalized)"="GenericSubVI", "Class Name (localized)"="GenericSubVI"}, "Class Heirarchy"="Generic.GObject.Node.SubVI.GenericSubVI", "Class Type"=enum."Scripting", "Indent"=4}, {"Class Info"={"Unique ID string"="16443", "Parent ID string"="16401", "Class Name (unlocalized)"="PolymorphicSubVI", "Class Name (localized)"="PolymorphicSubVI"}, "Class Heirarchy"="Generic.GObject.Node.SubVI.PolymorphicSubVI", "Class Type"=enum."Scripting", "Indent"=4}, {"Class Info"={"Unique ID string"="16540", "Parent ID string"="16421", "Class Name (unlocalized)"="TextBaseNode", "Class Name (localized)"="TextBaseNode"}, "Class Heirarchy"="Generic.GObject.Node.TextBaseNode", "Class Type"=enum."Scripting", "Indent"=3}, {"Class Info"={"Unique ID string"="16541", "Parent ID string"="16540", "Class Name (unlocalized)"="ExpressionNode", "Class Name (localized)"="ExpressionNode"}, "Class Heirarchy"="Generic.GObject.Node.TextBaseNode.ExpressionNode", "Class Type"=enum."Scripting", "Indent"=4}, {"Class Info"={"Unique ID string"="16403", "Parent ID string"="16421", "Class Name (unlocalized)"="UnitCast", "Class Name (localized)"="UnitCast"}, "Class Heirarchy"="Generic.GObject.Node.UnitCast", "Class Type"=enum."Scripting", "Indent"=3}, {"Class Info"={"Unique ID string"="16485", "Parent ID string"="16421", "Class Name (unlocalized)"="XNode", "Class Name (localized)"="XNode"}, "Class Heirarchy"="Generic.GObject.Node.XNode", "Class Type"=enum."Scripting", "Indent"=3}, {"Class Info"={"Unique ID string"="16497", "Parent ID string"="16485", "Class Name (unlocalized)"="XDataNode", "Class Name (localized)"="XDataNode"}, "Class Heirarchy"="Generic.GObject.Node.XNode.XDataNode", "Class Type"=enum."Scripting", "Indent"=4}, {"Class Info"={"Unique ID string"="75", "Parent ID string"="36", "Class Name (unlocalized)"="Pane", "Class Name (localized)"="Pane"}, "Class Heirarchy"="Generic.GObject.Pane", "Class Type"=enum."Base", "Indent"=2}, {"Class Info"={"Unique ID string"="31", "Parent ID string"="36", "Class Name (unlocalized)"="Panel", "Class Name (localized)"="Panel"}, "Class Heirarchy"="Generic.GObject.Panel", "Class Type"=enum."Base", "Indent"=2}, {"Class Info"={"Unique ID string"="16484", "Parent ID string"="36", "Class Name (unlocalized)"="PolymorphicVISelector", "Class Name (localized)"="PolymorphicVISelector"}, "Class Heirarchy"="Generic.GObject.PolymorphicVISelector", "Class Type"=enum."Scripting", "Indent"=2}, {"Class Info"={"Unique ID string"="16444", "Parent ID string"="36", "Class Name (unlocalized)"="PropertyItem", "Class Name (localized)"="PropertyItem"}, "Class Heirarchy"="Generic.GObject.PropertyItem", "Class Type"=enum."Scripting", "Indent"=2}, {"Class Info"={"Unique ID string"="40", "Parent ID string"="36", "Class Name (unlocalized)"="Scale", "Class Name (localized)"="Scale"}, "Class Heirarchy"="Generic.GObject.Scale", "Class Type"=enum."Base", "Indent"=2}, {"Class Info"={"Unique ID string"="43", "Parent ID string"="40", "Class Name (unlocalized)"="ColorGraphScale", "Class Name (localized)"="ColorGraphScale"}, "Class Heirarchy"="Generic.GObject.Scale.ColorGraphScale", "Class Type"=enum."Base", "Indent"=3}, {"Class Info"={"Unique ID string"="41", "Parent ID string"="40", "Class Name (unlocalized)"="ColorScale", "Class Name (localized)"="ColorScale"}, "Class Heirarchy"="Generic.GObject.Scale.ColorScale", "Class Type"=enum."Base", "Indent"=3}, {"Class Info"={"Unique ID string"="69", "Parent ID string"="41", "Class Name (unlocalized)"="RotaryColorScale", "Class Name (localized)"="RotaryColorScale"}, "Class Heirarchy"="Generic.GObject.Scale.ColorScale.RotaryColorScale", "Class Type"=enum."Base", "Indent"=4}, {"Class Info"={"Unique ID string"="42", "Parent ID string"="40", "Class Name (unlocalized)"="GraphScale", "Class Name (localized)"="GraphScale"}, "Class Heirarchy"="Generic.GObject.Scale.GraphScale", "Class Type"=enum."Base", "Indent"=3}, {"Class Info"={"Unique ID string"="52", "Parent ID string"="40", "Class Name (unlocalized)"="SlideScale", "Class Name (localized)"="SlideScale"}, "Class Heirarchy"="Generic.GObject.Scale.SlideScale", "Class Type"=enum."Base", "Indent"=3}, {"Class Info"={"Unique ID string"="16428", "Parent ID string"="36", "Class Name (unlocalized)"="SequenceLocal", "Class Name (localized)"="SequenceLocal"}, "Class Heirarchy"="Generic.GObject.SequenceLocal", "Class Type"=enum."Scripting", "Indent"=2}, {"Class Info"={"Unique ID string"="16475", "Parent ID string"="36", "Class Name (unlocalized)"="SimulationDCO", "Class Name (localized)"="SimulationDCO"}, "Class Heirarchy"="Generic.GObject.SimulationDCO", "Class Type"=enum."Scripting", "Indent"=2}, {"Class Info"={"Unique ID string"="76", "Parent ID string"="36", "Class Name (unlocalized)"="Splitter", "Class Name (localized)"="Splitter"}, "Class Heirarchy"="Generic.GObject.Splitter", "Class Type"=enum."Base", "Indent"=2}, {"Class Info"={"Unique ID string"="16491", "Parent ID string"="36", "Class Name (unlocalized)"="SynchronousDataFlowDCO", "Class Name (localized)"="SynchronousDataFlowDCO"}, "Class Heirarchy"="Generic.GObject.SynchronousDataFlowDCO", "Class Type"=enum."Scripting", "Indent"=2}, {"Class Info"={"Unique ID string"="16385", "Parent ID string"="36", "Class Name (unlocalized)"="Terminal", "Class Name (localized)"="Terminal"}, "Class Heirarchy"="Generic.GObject.Terminal", "Class Type"=enum."Scripting", "Indent"=2}, {"Class Info"={"Unique ID string"="16395", "Parent ID string"="16385", "Class Name (unlocalized)"="ControlTerminal", "Class Name (localized)"="ControlTerminal"}, "Class Heirarchy"="Generic.GObject.Terminal.ControlTerminal", "Class Type"=enum."Scripting", "Indent"=3}, {"Class Info"={"Unique ID string"="16441", "Parent ID string"="16385", "Class Name (unlocalized)"="InnerTerminal", "Class Name (localized)"="InnerTerminal"}, "Class Heirarchy"="Generic.GObject.Terminal.InnerTerminal", "Class Type"=enum."Scripting", "Indent"=3}, {"Class Info"={"Unique ID string"="16456", "Parent ID string"="16385", "Class Name (unlocalized)"="OuterTerminal", "Class Name (localized)"="OuterTerminal"}, "Class Heirarchy"="Generic.GObject.Terminal.OuterTerminal", "Class Type"=enum."Scripting", "Indent"=3}, {"Class Info"={"Unique ID string"="16514", "Parent ID string"="16385", "Class Name (unlocalized)"="ParameterTerminal", "Class Name (localized)"="ParameterTerminal"}, "Class Heirarchy"="Generic.GObject.Terminal.ParameterTerminal", "Class Type"=enum."Scripting", "Indent"=3}, {"Class Info"={"Unique ID string"="16515", "Parent ID string"="16514", "Class Name (unlocalized)"="OverridableParameterTerminal", "Class Name (localized)"="OverridableParameterTerminal"}, "Class Heirarchy"="Generic.GObject.Terminal.ParameterTerminal.OverridableParameterTerminal", "Class Type"=enum."Scripting", "Indent"=4}, {"Class Info"={"Unique ID string"="16493", "Parent ID string"="36", "Class Name (unlocalized)"="TimedStructDCO", "Class Name (localized)"="TimedStructDCO"}, "Class Heirarchy"="Generic.GObject.TimedStructDCO", "Class Type"=enum."Scripting", "Indent"=2}, {"Class Info"={"Unique ID string"="16426", "Parent ID string"="36", "Class Name (unlocalized)"="Tunnel", "Class Name (localized)"="Tunnel"}, "Class Heirarchy"="Generic.GObject.Tunnel", "Class Type"=enum."Scripting", "Indent"=2}, {"Class Info"={"Unique ID string"="16525", "Parent ID string"="16426", "Class Name (unlocalized)"="ConditionalTunnel", "Class Name (localized)"="ConditionalTunnel"}, "Class Heirarchy"="Generic.GObject.Tunnel.ConditionalTunnel", "Class Type"=enum."Scripting", "Indent"=3}, {"Class Info"={"Unique ID string"="16486", "Parent ID string"="16525", "Class Name (unlocalized)"="SelectorTunnel", "Class Name (localized)"="SelectorTunnel"}, "Class Heirarchy"="Generic.GObject.Tunnel.ConditionalTunnel.SelectorTunnel", "Class Type"=enum."Scripting", "Indent"=4}, {"Class Info"={"Unique ID string"="16442", "Parent ID string"="16426", "Class Name (unlocalized)"="LeftShiftRegister", "Class Name (localized)"="LeftShiftRegister"}, "Class Heirarchy"="Generic.GObject.Tunnel.LeftShiftRegister", "Class Type"=enum."Scripting", "Indent"=3}, {"Class Info"={"Unique ID string"="16427", "Parent ID string"="16426", "Class Name (unlocalized)"="LoopTunnel", "Class Name (localized)"="LoopTunnel"}, "Class Heirarchy"="Generic.GObject.Tunnel.LoopTunnel", "Class Type"=enum."Scripting", "Indent"=3}, {"Class Info"={"Unique ID string"="16536", "Parent ID string"="16426", "Class Name (unlocalized)"="RegionTunnel", "Class Name (localized)"="RegionTunnel"}, "Class Heirarchy"="Generic.GObject.Tunnel.RegionTunnel", "Class Type"=enum."Scripting", "Indent"=3}, {"Class Info"={"Unique ID string"="16399", "Parent ID string"="16426", "Class Name (unlocalized)"="RightShiftRegister", "Class Name (localized)"="RightShiftRegister"}, "Class Heirarchy"="Generic.GObject.Tunnel.RightShiftRegister", "Class Type"=enum."Scripting", "Indent"=3}, {"Class Info"={"Unique ID string"="16439", "Parent ID string"="36", "Class Name (unlocalized)"="Wire", "Class Name (localized)"="Wire"}, "Class Heirarchy"="Generic.GObject.Wire", "Class Type"=enum."Scripting", "Indent"=2}, {"Class Info"={"Unique ID string"="16454", "Parent ID string"="3", "Class Name (unlocalized)"="MasterWizard", "Class Name (localized)"="MasterWizard"}, "Class Heirarchy"="Generic.MasterWizard", "Class Type"=enum."Scripting", "Indent"=1}, {"Class Info"={"Unique ID string"="54", "Parent ID string"="3", "Class Name (unlocalized)"="Page", "Class Name (localized)"="Page"}, "Class Heirarchy"="Generic.Page", "Class Type"=enum."Base", "Indent"=1}, {"Class Info"={"Unique ID string"="37", "Parent ID string"="3", "Class Name (unlocalized)"="Plot", "Class Name (localized)"="Plot"}, "Class Heirarchy"="Generic.Plot", "Class Type"=enum."Base", "Indent"=1}, {"Class Info"={"Unique ID string"="16440", "Parent ID string"="3", "Class Name (unlocalized)"="Probe", "Class Name (localized)"="Probe"}, "Class Heirarchy"="Generic.Probe", "Class Type"=enum."Scripting", "Indent"=1}, {"Class Info"={"Unique ID string"="16463", "Parent ID string"="3", "Class Name (unlocalized)"="SubWizard", "Class Name (localized)"="SubWizard"}, "Class Heirarchy"="Generic.SubWizard", "Class Type"=enum."Scripting", "Indent"=1}, {"Class Info"={"Unique ID string"="16498", "Parent ID string"="16463", "Class Name (unlocalized)"="CodeWizard", "Class Name (localized)"="CodeWizard"}, "Class Heirarchy"="Generic.SubWizard.CodeWizard", "Class Type"=enum."Scripting", "Indent"=2}, {"Class Info"={"Unique ID string"="16547", "Parent ID string"="16463", "Class Name (unlocalized)"="ExternalEditorWizard", "Class Name (localized)"="ExternalEditorWizard"}, "Class Heirarchy"="Generic.SubWizard.ExternalEditorWizard", "Class Type"=enum."Scripting", "Indent"=2}, {"Class Info"={"Unique ID string"="16455", "Parent ID string"="16463", "Class Name (unlocalized)"="StateDiagramWizard", "Class Name (localized)"="StateDiagramWizard"}, "Class Heirarchy"="Generic.SubWizard.StateDiagramWizard", "Class Type"=enum."Scripting", "Indent"=2}, {"Class Info"={"Unique ID string"="91", "Parent ID string"="", "Class Name (unlocalized)"="LVTarget", "Class Name (localized)"="LVTarget"}, "Class Heirarchy"="LVTarget", "Class Type"=enum."Private", "Indent"=0}, {"Class Info"={"Unique ID string"="73", "Parent ID string"="", "Class Name (unlocalized)"="Project", "Class Name (localized)"="Project"}, "Class Heirarchy"="Project", "Class Type"=enum."Base", "Indent"=0}, {"Class Info"={"Unique ID string"="133", "Parent ID string"="", "Class Name (unlocalized)"="ProjectFilesViewItem", "Class Name (localized)"="ProjectFilesViewItem"}, "Class Heirarchy"="ProjectFilesViewItem", "Class Type"=enum."Private", "Indent"=0}, {"Class Info"={"Unique ID string"="74", "Parent ID string"="", "Class Name (unlocalized)"="ProjectItem", "Class Name (localized)"="ProjectItem"}, "Class Heirarchy"="ProjectItem", "Class Type"=enum."Base", "Indent"=0}, {"Class Info"={"Unique ID string"="77", "Parent ID string"="74", "Class Name (unlocalized)"="BuildSpecification", "Class Name (localized)"="BuildSpecification"}, "Class Heirarchy"="ProjectItem.BuildSpecification", "Class Type"=enum."Base", "Indent"=1}, {"Class Info"={"Unique ID string"="134", "Parent ID string"="74", "Class Name (unlocalized)"="LVClassPropDefFolder", "Class Name (localized)"="LVClassPropDefFolder"}, "Class Heirarchy"="ProjectItem.LVClassPropDefFolder", "Class Type"=enum."Base", "Indent"=1}, {"Class Info"={"Unique ID string"="80", "Parent ID string"="74", "Class Name (unlocalized)"="Library", "Class Name (localized)"="Library"}, "Class Heirarchy"="ProjectItem.Library", "Class Type"=enum."Base", "Indent"=1}, {"Class Info"={"Unique ID string"="85", "Parent ID string"="80", "Class Name (unlocalized)"="LVClassLibrary", "Class Name (localized)"="LVClassLibrary"}, "Class Heirarchy"="ProjectItem.Library.LVClassLibrary", "Class Type"=enum."Base", "Indent"=2}, {"Class Info"={"Unique ID string"="126", "Parent ID string"="80", "Class Name (unlocalized)"="StatechartLibrary", "Class Name (localized)"="StatechartLibrary"}, "Class Heirarchy"="ProjectItem.Library.StatechartLibrary", "Class Type"=enum."Base", "Indent"=2}, {"Class Info"={"Unique ID string"="103", "Parent ID string"="80", "Class Name (unlocalized)"="XInterfaceLibrary", "Class Name (localized)"="XInterfaceLibrary"}, "Class Heirarchy"="ProjectItem.Library.XInterfaceLibrary", "Class Type"=enum."Base", "Indent"=2}, {"Class Info"={"Unique ID string"="88", "Parent ID string"="103", "Class Name (unlocalized)"="XControlLibrary", "Class Name (localized)"="XControlLibrary"}, "Class Heirarchy"="ProjectItem.Library.XInterfaceLibrary.XControlLibrary", "Class Type"=enum."Base", "Indent"=3}, {"Class Info"={"Unique ID string"="89", "Parent ID string"="103", "Class Name (unlocalized)"="XNodeLibrary", "Class Name (localized)"="XNodeLibrary"}, "Class Heirarchy"="ProjectItem.Library.XInterfaceLibrary.XNodeLibrary", "Class Type"=enum."Base", "Indent"=3}, {"Class Info"={"Unique ID string"="125", "Parent ID string"="74", "Class Name (unlocalized)"="LibraryData", "Class Name (localized)"="LibraryData"}, "Class Heirarchy"="ProjectItem.LibraryData", "Class Type"=enum."Base", "Indent"=1}, {"Class Info"={"Unique ID string"="120", "Parent ID string"="74", "Class Name (unlocalized)"="PropertyFolder", "Class Name (localized)"="PropertyFolder"}, "Class Heirarchy"="ProjectItem.PropertyFolder", "Class Type"=enum."Base", "Indent"=1}, {"Class Info"={"Unique ID string"="119", "Parent ID string"="120", "Class Name (unlocalized)"="XPropertyFolder", "Class Name (localized)"="XPropertyFolder"}, "Class Heirarchy"="ProjectItem.PropertyFolder.XPropertyFolder", "Class Type"=enum."Base", "Indent"=2}, {"Class Info"={"Unique ID string"="95", "Parent ID string"="74", "Class Name (unlocalized)"="TargetItem", "Class Name (localized)"="TargetItem"}, "Class Heirarchy"="ProjectItem.TargetItem", "Class Type"=enum."Base", "Indent"=1}, {"Class Info"={"Unique ID string"="96", "Parent ID string"="", "Class Name (unlocalized)"="ProjectItemType", "Class Name (localized)"="ProjectItemType"}, "Class Heirarchy"="ProjectItemType", "Class Type"=enum."Private", "Indent"=0}, {"Class Info"={"Unique ID string"="93", "Parent ID string"="", "Class Name (unlocalized)"="Provider", "Class Name (localized)"="Provider"}, "Class Heirarchy"="Provider", "Class Type"=enum."Private", "Indent"=0}, {"Class Info"={"Unique ID string"="123", "Parent ID string"="", "Class Name (unlocalized)"="Scene", "Class Name (localized)"="Scene"}, "Class Heirarchy"="Scene", "Class Type"=enum."Base", "Indent"=0}, {"Class Info"={"Unique ID string"="128", "Parent ID string"="123", "Class Name (unlocalized)"="SceneDrawable", "Class Name (localized)"="SceneDrawable"}, "Class Heirarchy"="Scene.SceneDrawable", "Class Type"=enum."Base", "Indent"=1}, {"Class Info"={"Unique ID string"="112", "Parent ID string"="128", "Class Name (unlocalized)"="SceneGeometry", "Class Name (localized)"="SceneGeometry"}, "Class Heirarchy"="Scene.SceneDrawable.SceneGeometry", "Class Type"=enum."Base", "Indent"=2}, {"Class Info"={"Unique ID string"="113", "Parent ID string"="112", "Class Name (unlocalized)"="SceneBox", "Class Name (localized)"="SceneBox"}, "Class Heirarchy"="Scene.SceneDrawable.SceneGeometry.SceneBox", "Class Type"=enum."Base", "Indent"=3}, {"Class Info"={"Unique ID string"="114", "Parent ID string"="112", "Class Name (unlocalized)"="SceneCone", "Class Name (localized)"="SceneCone"}, "Class Heirarchy"="Scene.SceneDrawable.SceneGeometry.SceneCone", "Class Type"=enum."Base", "Indent"=3}, {"Class Info"={"Unique ID string"="115", "Parent ID string"="112", "Class Name (unlocalized)"="SceneCylinder", "Class Name (localized)"="SceneCylinder"}, "Class Heirarchy"="Scene.SceneDrawable.SceneGeometry.SceneCylinder", "Class Type"=enum."Base", "Indent"=3}, {"Class Info"={"Unique ID string"="116", "Parent ID string"="112", "Class Name (unlocalized)"="SceneHeightField", "Class Name (localized)"="SceneHeightField"}, "Class Heirarchy"="Scene.SceneDrawable.SceneGeometry.SceneHeightField", "Class Type"=enum."Base", "Indent"=3}, {"Class Info"={"Unique ID string"="118", "Parent ID string"="112", "Class Name (unlocalized)"="SceneMesh", "Class Name (localized)"="SceneMesh"}, "Class Heirarchy"="Scene.SceneDrawable.SceneGeometry.SceneMesh", "Class Type"=enum."Base", "Indent"=3}, {"Class Info"={"Unique ID string"="117", "Parent ID string"="112", "Class Name (unlocalized)"="SceneSphere", "Class Name (localized)"="SceneSphere"}, "Class Heirarchy"="Scene.SceneDrawable.SceneGeometry.SceneSphere", "Class Type"=enum."Base", "Indent"=3}, {"Class Info"={"Unique ID string"="129", "Parent ID string"="128", "Class Name (unlocalized)"="SceneText", "Class Name (localized)"="SceneText"}, "Class Heirarchy"="Scene.SceneDrawable.SceneText", "Class Type"=enum."Base", "Indent"=2}, {"Class Info"={"Unique ID string"="104", "Parent ID string"="123", "Class Name (unlocalized)"="SceneNode", "Class Name (localized)"="SceneNode"}, "Class Heirarchy"="Scene.SceneNode", "Class Type"=enum."Base", "Indent"=1}, {"Class Info"={"Unique ID string"="110", "Parent ID string"="104", "Class Name (unlocalized)"="SceneClipPlane", "Class Name (localized)"="SceneClipPlane"}, "Class Heirarchy"="Scene.SceneNode.SceneClipPlane", "Class Type"=enum."Base", "Indent"=2}, {"Class Info"={"Unique ID string"="106", "Parent ID string"="104", "Class Name (unlocalized)"="SceneLight", "Class Name (localized)"="SceneLight"}, "Class Heirarchy"="Scene.SceneNode.SceneLight", "Class Type"=enum."Base", "Indent"=2}, {"Class Info"={"Unique ID string"="105", "Parent ID string"="104", "Class Name (unlocalized)"="SceneObject", "Class Name (localized)"="SceneObject"}, "Class Heirarchy"="Scene.SceneNode.SceneObject", "Class Type"=enum."Base", "Indent"=2}, {"Class Info"={"Unique ID string"="111", "Parent ID string"="123", "Class Name (unlocalized)"="SceneTexture", "Class Name (localized)"="SceneTexture"}, "Class Heirarchy"="Scene.SceneTexture", "Class Type"=enum."Base", "Indent"=1}, {"Class Info"={"Unique ID string"="84", "Parent ID string"="123", "Class Name (unlocalized)"="SceneWindow", "Class Name (localized)"="SceneWindow"}, "Class Heirarchy"="Scene.SceneWindow", "Class Type"=enum."Base", "Indent"=1}, {"Class Info"={"Unique ID string"="82", "Parent ID string"="", "Class Name (unlocalized)"="TagSet", "Class Name (localized)"="TagSet"}, "Class Heirarchy"="TagSet", "Class Type"=enum."Private", "Indent"=0}, {"Class Info"={"Unique ID string"="2", "Parent ID string"="", "Class Name (unlocalized)"="VI", "Class Name (localized)"="VI"}, "Class Heirarchy"="VI", "Class Type"=enum."Base", "Indent"=0}, {"Class Info"={"Unique ID string"="79", "Parent ID string"="2", "Class Name (unlocalized)"="FacadeVI", "Class Name (localized)"="FacadeVI"}, "Class Heirarchy"="VI.FacadeVI", "Class Type"=enum."Base", "Indent"=1}, {"Class Info"={"Unique ID string"="87", "Parent ID string"="2", "Class Name (unlocalized)"="MethodVI", "Class Name (localized)"="MethodVI"}, "Class Heirarchy"="VI.MethodVI", "Class Type"=enum."Base", "Indent"=1}, {"Class Info"={"Unique ID string"="101", "Parent ID string"="2", "Class Name (unlocalized)"="PolymorphicVI", "Class Name (localized)"="PolymorphicVI"}, "Class Heirarchy"="VI.PolymorphicVI", "Class Type"=enum."Base", "Indent"=1}, {"Class Info"={"Unique ID string"="62", "Parent ID string"="2", "Class Name (unlocalized)"="SubsystemVI", "Class Name (localized)"="SubsystemVI"}, "Class Heirarchy"="VI.SubsystemVI", "Class Type"=enum."Base", "Indent"=1}, {"Class Info"={"Unique ID string"="81", "Parent ID string"="", "Class Name (unlocalized)"="Variable", "Class Name (localized)"="Variable"}, "Class Heirarchy"="Variable", "Class Type"=enum."Base", "Indent"=0}]) -> (0 "Error Out":errorcluster, 3 "Unique ID of Selected Item":string[](array[string]))   [LabVIEW 2023]
doc: "Dialog to select items from the input cluster ref. \n\nFilter narrows list of items.\nDown key puts focus on tree and selects first item.\nUp and Down keps navigate tree.\nMultiple items can be selected.\n\nIn case of action \"Delete\" (\"Remove elements(s)...\" selected), list will show all elements currently displayed, else it will show all elements availabel to undle or unbundle.\n\nOutput is a list of the selected item tags."
uses:
  <userlib>/_OpenG.lib/error/error.llb/openg_error.lvlib
  controls/action enum.ctl
  <userlib>/_OpenG.lib/appcontrol/appcontrol.llb/openg_application_control.lvlib
  controls/Done Button.ctl
panel:
  in  "Filter":string
  in  "Tree":string[](tree)
  in  "Show":T1
  in  "Done":T2
  # "Debug"
  # "All panes scroll to origin at runtime, so we don't have to worry about pane placements\n\nThis pane contracts at runtime and vertical splitter to left sticks to right at runtime so resizing functions happen as expected."
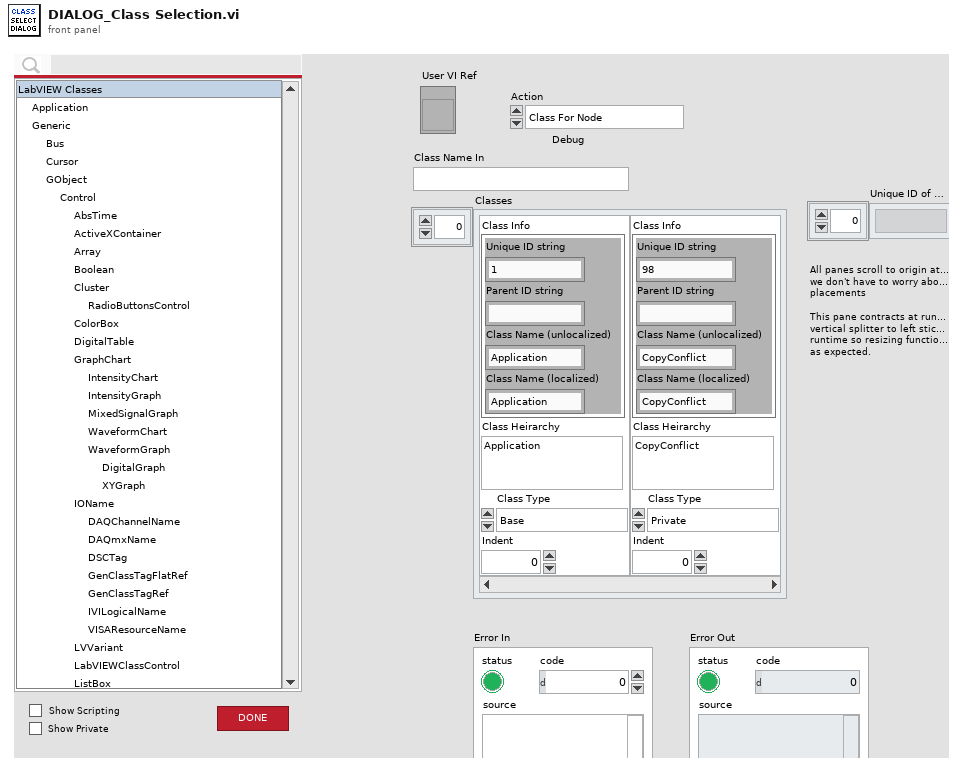
[diagram p1: front panel]
types:
  T1 = cluster{"Show Scripting":bool, "Show Private":bool}
  T2 = typedef "Done Button.ctl" = bool
  T3 = typedef "action enum.ctl" = enum16{"[NONE]", "APP_SEPARATOR", "Wire Bundle", "Wire Unbundle", "Terminal Unbundle", "Terminal Bundle", "Bundler Move Up", "Bundler Move Down", "Bundler Insert", "Bundler Remove", "Bundler Remove Unwired", "Bundler Rearrange", "In Place Insert", "In Place Remove", "In Place Remove Unwired", "In Place Rearrange", "Wire Properties", "Wire Method", "Terminal Properties", "Terminal Method", "Property Move Up", "Property Move Down", "Properties Insert", "Properties Remove", "Properties Remove Unwired", "Properties Rearrange", "Method Change", "Class For Constant", "Class For Control", "Class For Node", "Class Name to Clipboard"}
  T4 = cluster{"Class Info":cluster{"Unique ID string":string, "Parent ID string":string, "Class Name (unlocalized)":string, "Class Name (localized)":string}, "Class Heirarchy":string, "Class Type":enum16{"Unknown", "Base", "Scripting", "Private", "Deprecated", "None", "Divider"}, "Indent":u32}[]
  T5 = typedef "Class Item Cluster.ctl" = cluster{"Tree Item":cluster{"Left Cell String":string, "Child Text":string[], "Child Tag":string, "Item Indent":i32, "Child Only?":bool, "Glyph Index":i32}, "Disabled?":bool, "Nest Chain":string[]}
  T6 = typedef "eventvkey.ctl" = enum16{"ASCII", "Enter", "Return", "Shift", "Ctrl", "Alt", "Cmd", "Opt", "Caps", "NumLock", "Clear", "Break", "Up", "Down", "Left", "Right", "Insert", "Delete", "Home", "End", "PageUp", "PageDown", "Escape", "Help", "Pause", "ScrollLock", "F1", "F2", "F3", "F4", "F5", "F6", "F7", "F8", "F9", "F10", "F11", "F12", "F13", "F14", "F15", "F16", "F17", "F18", "F19", "F20", "F21", "F22", "F23", "F24", "Play", "VolumeUp", "VolumeDown", "Mute", "Two Byte Char"}
  T7 = cluster{"Index":u16, "Property Type":enum16{"Unknown", "Base", "Scripting", "Private", "Deprecated", "None", "Divider"}, "ID String":string, "Dotted ID String":string, "Class":string, "Parent":string, "Display name full":string, "Display name short":string, "Parents Array":string[], "Indent":u16}
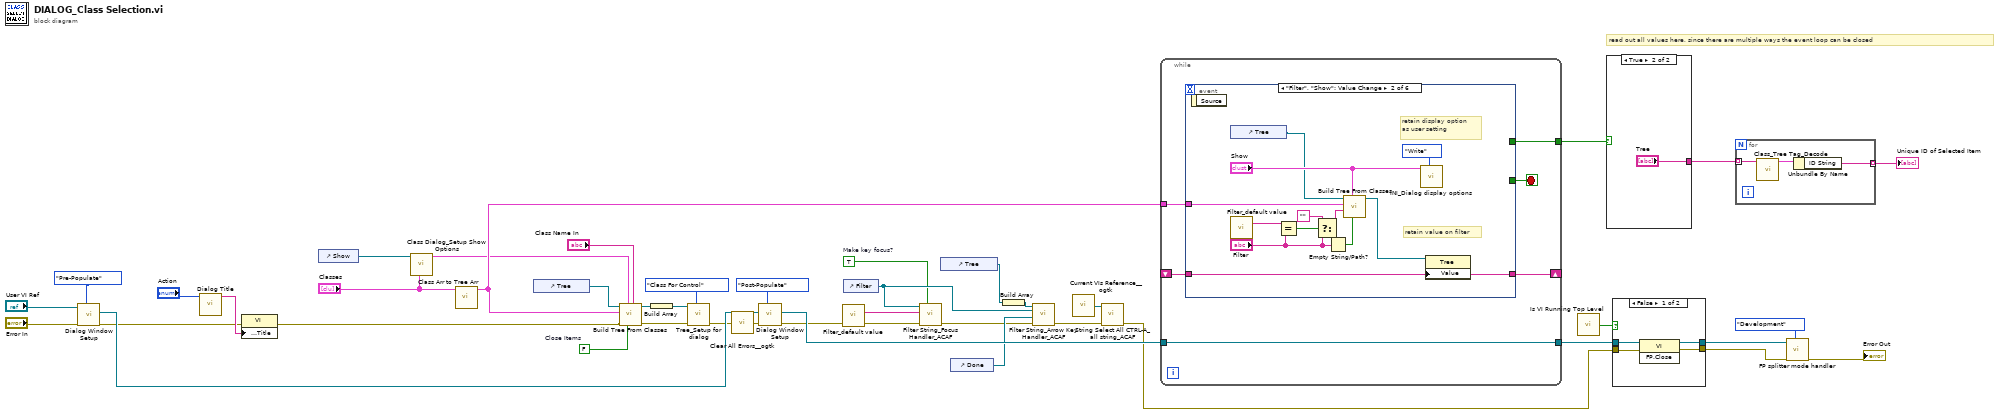
[diagram p0: block diagram]
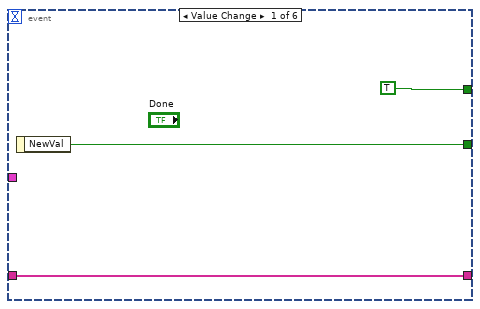
[diagram p2: hidden frame]
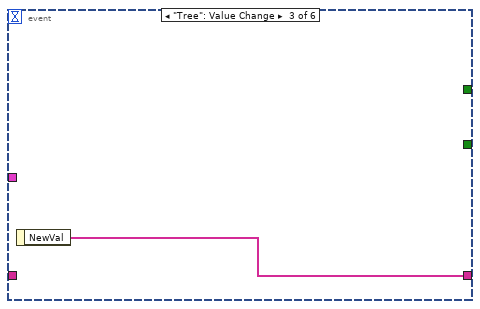
[diagram p3: hidden frame]
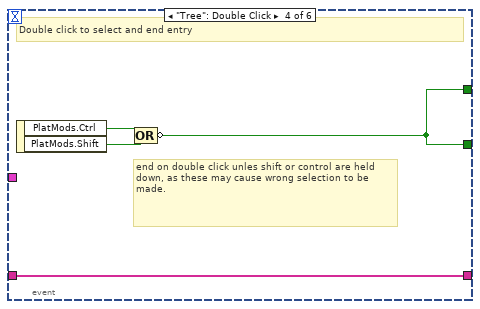
[diagram p4: hidden frame]
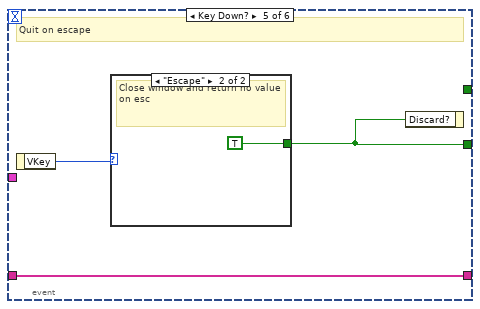
[diagram p5: hidden frame]
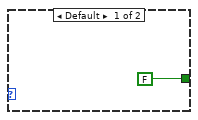
[diagram p6: hidden frame]
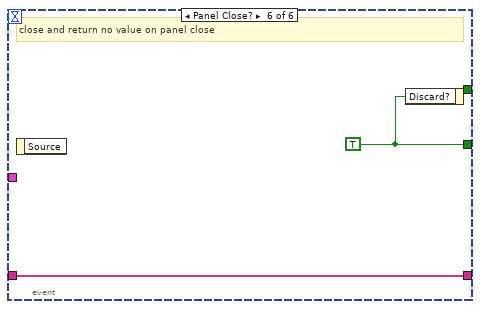
[diagram p7: hidden frame]
diagram:
  w2 = TRUE  # Make key focus?
  w25 = FALSE  # Close Items
  # "read out all values here, since there are multiple ways the event loop can be closed"
  n1 = call "Dialog Window Setup.vi"("Action"=enum16{"Pre-Populate", "Post-Populate"}."Pre-Populate", "error in"="Error In", "Align-to Window Ref"="User VI Ref") -> ("error out"=w8:errorcluster, "Dialog VI Ref Out"=w29:refnum<vi>)  [unwired: 7 in]
  n2 = call "Dialog Title.vi"("Action"="Action") -> ("Window Title"=w11:string)  [unwired: 10 in]
  n3 = property class="VI"(error in=w8, "Front Panel.Title"=w11) -> (error out=w7:errorcluster)  [unwired: 1 in, 1 out]
  n4 = control-ref of="Show"() -> (w12:refnum<vi>)
  n5 = call "Class Dialog_Setup Show Options.vi"("Classes"="Classes", "Cluster in"=w12) -> ("Display Options Out"=w23:T1)  [unwired: 9 in]
  n6 = call "Class Arr to Tree Arr.vi"("Sorted Classes"="Classes") -> ("Array"=w34:T5[])  [unwired: 10 in]
  n7 = control-ref of="Tree"() -> (w24:refnum<vi>)
  n8 = call "Build Tree From Classes.vi"("Selected Item (None)"="Class Name In", "Close Items"=w25, "Show"=w23, "error in"=w7, "Class Tree Array"=w34, "Tree Ref"=w24) -> ("error out"=w37:errorcluster, "Tree Ref Out"=w36:refnum<vi>)  [unwired: 4 in]
  n9 = Build Array(w36) -> (w35:refnum<vi>[])
  n10 = call "Tree_Setup for dialog.vi"("Action"=action_enum."Class For Control", "error in"=w37, "Tree Ref"=w35) -> ("error out"=w28:errorcluster)  [unwired: 7 in, 1 out]
  n11 = call <userlib>:"Clear All Errors__ogtk.vi"("Error In"=w28) -> ("Error Out"=w26:errorcluster)  [unwired: 3 in]
  n12 = call "Dialog Window Setup.vi"("Action"=enum16{"Pre-Populate", "Post-Populate"}."Post-Populate", "error in"=w26, "Dialog VI Ref In [Parent]"=w29) -> ("error out"=w6:errorcluster, "Dialog VI Ref Out"=w27:refnum<vi>)  [unwired: 7 in]
  n13 = call "Filter_default value.vi"() -> ("Filter Default Value"=w4:string)  [unwired: 3 in]
  n14 = control-ref of="Filter"() -> (w3:refnum<vi>)
  n15 = call "Filter String_Focus Handler_ACAF.vi"("Make key focus?"=w2, "error in (no error)"=w6, "Default Value"=w4, "Filter String Ref"=w3) -> ("error out"=w5:errorcluster)  [unwired: 7 in]
  n16 = control-ref of="Tree"() -> (w15:refnum<vi>)
  n17 = control-ref of="Done"() -> (w14:refnum<vi>)
  n18 = Build Array(w15) -> (w16:refnum<vi>[])
  n19 = call "Filter String_Arrow Key Handler_ACAF.vi"("error in (no error)"=w5, "Done Ref"=w14, "Filter String Ref"=w3, "Tree Ref Array"=w16) -> ()  [unwired: 7 in, 1 out]
  n20 = call <userlib>:"Current VIs Reference__ogtk.vi"() -> ("Current VI's reference"=w18:refnum<vi>)  [unwired: 5 in]
  n21 = call "String Select All CTRL-A_all string_ACAF.vi"("error in (no error)"=w5, "VI Ref"=w18) -> ("error out"=w17:errorcluster)  [unwired: 9 in]
  n22 = while {
    tunnel: [w47] -> w42
    tunnel: [w46] -> w40
    tunnel: w27 -> [w46]
    tunnel: w34 -> [w45]
    shift-right: [w44] -> _
    shift-left: _ -> [w43]
    stop <- w48 stop-if-true
    n23 = event shown="[1] \"Filter\", \"Show\": Value Change" {
      selector: _ -> [_ _ _ _ _ _]
      dyn-events: _ -> [_ _ _ _ _ _]
      timeout: _ -> [_ _ _ _ _ _]
      tunnel: [w51 _ _ w66 w70 w75] -> w48
      tunnel: [TRUE _ _ w66 _ _] -> w47
      tunnel: w45 -> [_ w63 _ _ _ _]
      tunnel: [w49 w58 w64 w65 w69 w74] -> w44
      tunnel: w43 -> [w49 w58 _ w65 w69 w74]
      event Value Change {
        n24 = event-data() -> ("NewVal"=w51:T2)  [unwired: 1 in]
      }
      event "Filter", "Show": Value Change {
        # "retain display option as user setting"
        # "retain value on filter"
        n25 = event-data() -> ()  [unwired: 1 in, 1 out]
        n26 = control-ref of="Tree"() -> (w52:refnum<vi>)
        n27 = call "Filter_default value.vi"() -> ("Filter Default Value"=w53:string)  [unwired: 3 in]
        n28 = Equal?(x=w53, y="Filter") -> (x = y?=w62:bool)
        n29 = Select(t="", s=w62, f="Filter") -> (s? t:f=w61:string)
        n30 = Empty String/Path?(string/path="Filter") -> (empty?=w54:bool)
        n31 = call "Build Tree From Classes.vi"("Close Items"=w54, "Show"="Show", "Filter"=w61, "Class Tree Array"=w63, "Tree Ref"=w52) -> ("Tree Ref Out"=w59:refnum<vi>)  [unwired: 5 in, 1 out]
        n32 = call "INI_Dialog display options.vi"("File Action"=enum16{"Read", "Write"}."Write", "Display Options"="Show") -> ()  [unwired: 9 in, 1 out]
        n33 = property class="Tree"(reference=w59, "Value"=w58) -> ()  [unwired: 1 in, 2 out]
      }
      event "Tree": Value Change {
        n34 = event-data() -> ("NewVal"=w64:string[])  [unwired: 1 in]
      }
      event "Tree": Double Click {
        # "end on double click unles shift or control are held down, as these may cause wrong selection to be made."
        # "Double click to select and end entry"
        n35 = event-data() -> ("PlatMods.Ctrl"=w68:bool, "PlatMods.Shift"=w67:bool)  [unwired: 1 in]
        n36 = Compound Arithmetic op=OR(w68, w67) -> (invert w66:bool)
      }
      event Key Down? {
        # "Quit on escape"
        n37 = event-data() -> ("VKey"=w71:T6)  [unwired: 1 in]
        n38 = case shown="\"Escape\"" w71 {
          tunnel: [FALSE TRUE] -> w70
          frame Default {
          }
          frame "Escape" {
            # "Close window and return no value on esc"
          }
        }
        n39 = event-data("Discard?"=w70) -> ()  [unwired: 1 in, 1 out]
      }
      event Panel Close? {
        w75 = TRUE
        # "close and return no value on panel close"
        n40 = event-data() -> ()  [unwired: 1 in, 1 out]
        n41 = event-data("Discard?"=w75) -> ()  [unwired: 1 in, 1 out]
      }
    }
  }
  n42 = call "Is VI Running Top Level.vi"() -> ("Top Level?"=w38:bool)  [unwired: 5 in]
  n43 = case shown="True" w42 {
    tunnel: [_ "Tree"] -> w32
    frame False {
    }
    frame True {
    }
  }
  n44 = case shown="False" w38 {
    tunnel: w40 -> [w80 w82]
    tunnel: [w79 w82] -> w39
    tunnel: w17 -> [w78 w81]
    tunnel: [w77 w81] -> w21
    frame False {
      n45 = invoke class="VI" method="FP.Close"(reference=w80, error in=w78) -> (reference out=w79:refnum<vi>, error out=w77:errorcluster)  [unwired: 1 in, 1 out]
    }
    frame True {
    }
  }
  n46 = for {
    tunnel: w32 -> [w85] mode=indexing
    tunnel: [w83] -> w19 mode=indexing
    n47 = call "Class_Tree Tag_Decode.vi"("Tag In"=w85) -> ("TagData"=w84:T7)  [unwired: 10 in]
    n48 = Unbundle By Name(w84) -> ("ID String"=w83:string)
  }
  "Unique ID of Selected Item" <- w19
  n49 = call "FP splitter mode handler.vi"("Mode"=enum16{"Run", "Development"}."Development", "error in"=w21, "VI Ref In"=w39) -> ("error out"=→"Error Out":errorcluster)  [unwired: 7 in, 1 out]
